vi "FL24 Combi Tool Main.vi"() -> ()   [LabVIEW 2016]
uses:
  Common/LabVIEW GEA2 Toolkit/LabVIEW_GEA2_Toolkit.lvlibp/type defs/Data In.ctl
  Common/LabVIEW GEA2 Toolkit/LabVIEW_GEA2_Toolkit.lvlibp/type defs/Source_Destination.ctl
  Common/LabVIEW GEA2 Toolkit/LabVIEW_GEA2_Toolkit.lvlibp/type defs/Data Type.ctl
  Common/LabVIEW GEA2 Toolkit/LabVIEW_GEA2_Toolkit.lvlibp/type defs/ERD Read Data In.ctl
  Laundry Tool 2.0 Support/type defs2/Select _Graph_Brass.ctl
  Laundry Tool 1.0 Support/type defs/ERD_Graph_All.ctl
  Laundry Tool 1.0 Support/type defs/ERD_Graph.ctl
  Laundry Tool 1.0 Support/type defs/Version.ctl
  Laundry Tool 2.0 Support/type defs2/ERD_Always_Show_Brass.ctl
  Laundry Tool 1.0 Support/type defs/Fault_Buffer_Status.ctl
  Laundry Tool 2.0 Support/type defs2/Diagnostics_Table.ctl
  Laundry Tool 1.0 Support/type defs/Cycle_Diag_Buffer_Status.ctl
  Laundry Tool 1.0 Support/type defs/Motor Control.ctl
  Laundry Tool 1.0 Support/type defs/Valves.ctl
  Laundry Tool 2.0 Support/type defs2/Programming_Brass.ctl
  Laundry Tool 2.0 Support/type defs2/Flash_Results.ctl
  Laundry Tool 2.0 Support/type defs2/ERD_Data_Loop_Control_Brass.ctl
  Laundry Tool 2.0 Support/type defs2/ERD_Loop_States_Brass.ctl
  Laundry Tool 2.0 Support/type defs2/DAQ_States_Brass.ctl
  Laundry Tool 2.0 Support/type defs2/Error_Command_Brass.ctl
  Common/GExplorer Support/typedefs/GExplorer_Data_Cluster.ctl
  Laundry Tool 1.0 Support/type defs/Cont_Send_States.ctl
  Laundry Tool 2.0 Support/type defs2/Cont_Send_States_Brass.ctl
  Common/LabVIEW GEA2 Toolkit/LabVIEW_GEA2_Toolkit.lvlibp/type defs/Data Out.ctl
  Common/LabVIEW GEA2 Toolkit/LabVIEW_GEA2_Toolkit.lvlibp/type defs/ERD Write Data In.ctl
  Laundry Tool 2.0 Support/type defs2/ERD_Loop_Control_Command_Brass.ctl
  Laundry Tool 2.0 Support/type defs2/GEA2_Control_Command_Brass.ctl
  Common/LabVIEW GEA2 Toolkit/LabVIEW_GEA2_Toolkit.lvlibp/advanced/GEA2 Message Received Event Handler.vi
  C:/Automation/DLLs/PC Dot Net/GeaCommunication.dll
  Automation/DLLs/PC Dot Net/GeaCommunication.dll
  Common/LabVIEW GEA2 Toolkit/LabVIEW_GEA2_Toolkit.lvlibp
panel:
  in  "Data ON":bool=TRUE
  out "ERD_Always Show":T1
  in  "Stop":bool
  out "Fault Status":bool
  out "Log Rate (ms)":u32
  in  "Tab Control":T2(tab)
  in  "Programming":T3={"Program"=FALSE, "File Path"=path "", "Program Ind"=FALSE, "Result"=9, "Reset Board"=FALSE, "Enter Bootloader"=FALSE} {"Result" items=["ImageRejected", "BoardNotFound", "UnableToGetGeaConfiguration", "WriteToFlashNotAllowed", "ImageDownloadedSuccessfully", "ImagePresent", "WriteToFlashFailed", "EraseFailed", "CrcFailed", ""]}
  in  "Filter Data":bool=TRUE
  in  "Start Send":bool
  in  "Cmd":string
  in  "Filter Log":bool
  in  "Msg Rate (ms)":u32=1000 min=50 step=50
  out "CSV File Log Path":path=path "C:/Users/502129737/Desktop/1"
  in  "Clear":bool
  out "GEA2 Log":string
  in  "Board Index":u8 max=0 step=1
  out "Board ID":string="0"
  in  "GEA2 Send":T5={"Source"=228, "Destination"=60, "Command"=0, "Message"=""} {"Command" format="%02x"; "Destination" format="%02x"; "Source" format="%02x"}
  in  "Send Button":bool
  in  "GEA2 Log Length":i32=100000
  in  "Save Log":bool
  out "Version":T6
  in  "GEA Inputs":T7={"Source"=228, "Destination"=60} {"Destination" format="%.0x"; "Source" format="%.0x"}
  in  "Read ERD List":T8[](array[typedef])=[{"ERD Number"=0, "Data Type"=enum."string"}] {"ERD Number" format="%.0x"}
  out "Read ERD Data Out":cluster{"ERD Number":u16, "Data":string}[](array[cluster]) {"ERD Number" format="%.0x"}
  in  "Read ERD":bool
  in  "Write ERD":bool
  in  "Write ERD List":T10(array[cluster])=[{"ERD Number"=0, "Data Type"=enum."string", "Data"=""}] {"ERD Number" format="%.0x"}
  out "Washer Loads":u16[][](graph)=[[0, 100, 200, 300, 400]]
  in  "ERD Graphing ON":bool
  out "ERD Graph  Ind":T11
  in  "ERD Graph Cntrl":T12={"ERD 3"={"ERD #"=61458, "Data Type"=enum."uint16_t", "Scaler"=100}, "ERD 2"={"ERD #"=61458, "Data Type"=enum."uint16_t", "Scaler"=100}, "ERD 1"={"ERD #"=61458, "Data Type"=enum."uint16_t", "Scaler"=100}} {"ERD 1"."Scaler" min=1; "ERD 1"."ERD #" format="%.0x"; "ERD 2"."Scaler" min=1; "ERD 2"."ERD #" format="%.0x"; "ERD 3"."Scaler" min=1; "ERD 3"."ERD #" format="%.0x"}
  in  "Graphing ON":bool=TRUE
  in  "Select Graph":T14
  out "ERD 3":dbl(graph)
  out "ERD 2":dbl(graph)
  out "ERD 1":dbl(graph)
  out "Water Temperature":dbl(graph)
  out "Basket Speed":u16(graph)
  out "Pressure 2":dbl(graph)
  out "Dryer Loads":dbl[][](graph)
  in  "Save Fault Log":bool
  in  "Clear Fault Table Buffer":bool
  in  "Clear Fault Seq Buffer":bool
  in  "Fault ON":bool
  out "Fault Table Buffer":string[][](table)
  out "Fault Sequence Buffer":string
  out "Seq Buffer Status":T15
  out "Table Buffer Status":T15
  in  "Save Cycle History Log":bool
  in  "Clear Cycle Buffer":bool
  out "Cycle Buffer Status":T16
  in  "Get Cycle History":bool
  out "Diagnostics Table":T17
  in  "Buzzer":cluster{"Test":bool}
  in  "Drain Pump":cluster{"ON":bool, "OFF":bool}
  in  "Valve Control":T18
  in  "Motor Control":T19={"Speed (RPM)"=50, "Start Motor"=FALSE, "Stop Motor"=FALSE} {"Speed (RPM)" min=-100 max=1400 step=50}
  in  "Test Mode":cluster{"Exit":bool, "Enter":bool}
  in  "Door Lock":cluster{"Lock Door":bool, "Unlock Door":bool}
  in  "LEDs":cluster{"ON":bool, "OFF":bool}
  in  "Drum Light":cluster{"ON":bool, "OFF":bool}
  in  "Water Heater":cluster{"ON":bool, "OFF":bool}
  in  "Dry Heater":cluster{"ON":bool, "OFF":bool}
  in  "ERD Read List":T20(array[cluster])=[{"Boolean"=TRUE, "ERD Number"=1, "ERD Name"="Model Number", "Data Type"=enum."string"}, {"Boolean"=TRUE, "ERD Number"=2, "ERD Name"="Serial Number", "Data Type"=enum."string"}, {"Boolean"=TRUE, "ERD Number"=8192, "ERD Name"="Machine Status", "Data Type"=enum."uint8_t"}, {"Boolean"=TRUE, "ERD Number"=8202, "ERD Name"="Cycle Name", "Data Type"=enum."string"}, {"Boolean"=TRUE, "ERD Number"=8213, "ERD Name"="Soil Level", "Data Type"=enum."string"}, {"Boolean"=TRUE, "ERD Number"=142, "ERD Name"="Cycle Count", "Data Type"=enum."uint32_t"}, {"Boolean"=TRUE, "ERD Number"=8193, "ERD Name"="Sub-Cycle", "Data Type"=enum."string"}, {"Boolean"=TRUE, "ERD Number"=141, "ERD Name"="System Runtime", "Data Type"=enum."uint32_t"}, {"Boolean"=TRUE, "ERD Number"=8208, "ERD Name"="Delay Time", "Data Type"=enum."uint16_t"}, {"Boolean"=TRUE, "ERD Number"=70, "ERD Name"="Cycle Time", "Data Type"=enum."uint16_t"}, {"Boolean"=TRUE, "ERD Number"=8206, "ERD Name"="Operating Mode", "Data Type"=enum."string"}, {"Boolean"=TRUE, "ERD Number"=8214, "ERD Name"="Temp Level", "Data Type"=enum."uint8_t"}, {"Boolean"=TRUE, "ERD Number"=8215, "ERD Name"="Spin Level", "Data Type"=enum."uint8_t"}, {"Boolean"=TRUE, "ERD Number"=61440, "ERD Name"="Water Level", "Data Type"=enum."uint8_t"}, {"Boolean"=TRUE, "ERD Number"=8216, "ERD Name"="Rinse Option", "Data Type"=enum."uint8_t"}, {"Boolean"=TRUE, "ERD Number"=4, "ERD Name"="Control Lock", "Data Type"=enum."string"}, {"Boolean"=TRUE, "ERD Number"=10, "ERD Name"="Signal Volume", "Data Type"=enum."string"}, {"Boolean"=TRUE, "ERD Number"=8236, "ERD Name"="Basket Speed", "Data Type"=enum."uint16_t"}, {"Boolean"=TRUE, "ERD Number"=8210, "ERD Name"="Door Status", "Data Type"=enum."string"}, {"Boolean"=TRUE, "ERD Number"=8211, "ERD Name"="Lock Status", "Data Type"=enum."string"}, {"Boolean"=TRUE, "ERD Number"=8258, "ERD Name"="Pressure (inches)", "Data Type"=enum."uint32_t"}, {"Boolean"=TRUE, "ERD Number"=8259, "ERD Name"="Water Temperature", "Data Type"=enum."uint16_t"}, {"Boolean"=TRUE, "ERD Number"=61458, "ERD Name"="Pressure Hz", "Data Type"=enum."uint16_t"}, {"Boolean"=TRUE, "ERD Number"=61455, "ERD Name"="Load Status 2", "Data Type"=enum."uint8_t"}, {"Boolean"=TRUE, "ERD Number"=61456, "ERD Name"="Load Status 1", "Data Type"=enum."uint8_t"}, {"Boolean"=TRUE, "ERD Number"=61460, "ERD Name"="Firmware Version", "Data Type"=enum."string"}, {"Boolean"=TRUE, "ERD Number"=61452, "ERD Name"="Drum Light", "Data Type"=enum."string"}, {"Boolean"=TRUE, "ERD Number"=14, "ERD Name"="Voltage", "Data Type"=enum."uint16_t"}, {"Boolean"=TRUE, "ERD Number"=61461, "ERD Name"="Inlet Thermistor", "Data Type"=enum."uint16_t"}, {"Boolean"=TRUE, "ERD Number"=61462, "ERD Name"="Outlet Themistor", "Data Type"=enum."uint16_t"}, {"Boolean"=TRUE, "ERD Number"=8275, "ERD Name"="Extended Tumble", "Data Type"=enum."string"}, {"Boolean"=TRUE, "ERD Number"=8277, "ERD Name"="Time Saver", "Data Type"=enum."string"}] {"ERD Number" format="%.0x"}
  out "Error Out":errorcluster
  in  "Error In":errorcluster
  # "UI: 0x3C\nMC: 0x21"
  # "Software Version"
  # "UI - Critical Version"
  # "UI - Non-Critical"
  # "MC -  Version"
  # "Inverter Version"
  # "Model Setting"
  # "Must input a valid ERD# and Data Type\nDO NOT Leave Blank \nIf no scaler use value of 01"
  # "+ CCW   - CW"
  # "Contact:\n\nDerek Hibdon\nderek.hibdon@ge.com"
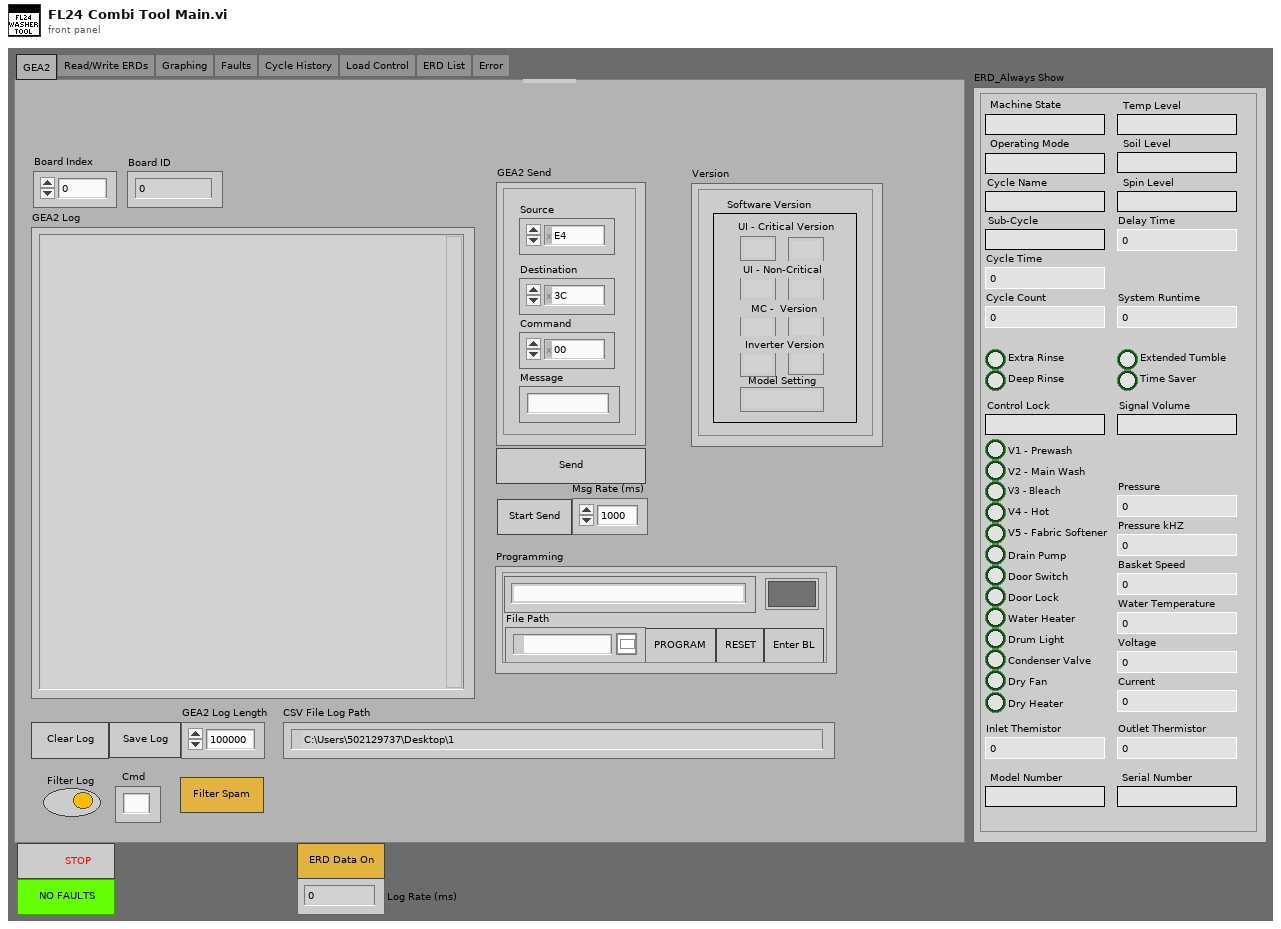
[diagram p1: front panel]
types:
  T1 = typedef "ERD_Always_Show_Brass.ctl" = cluster{"Machine State":string, "Cycle Count":u32, "Soil Level":string, "Spin Level":string, "Temp Level":string, "Delay Time":u16, "Sub-Cycle":string, "Cycle Name":string, "Model Number":string, "Serial Number":string, "System Runtime":u32, "Cycle Time":u16, "Operating Mode":string, "Deep Rinse":bool, "Extra Rinse":bool, "V1 - Prewash":bool, "V2 - Main Wash":bool, "V3 - Bleach":bool, "V4 - Hot":bool, "Drain Pump":bool, "Door Switch":bool, "Door Lock":bool, "Basket Speed":u16, "Water Temperature":dbl, "Voltage":dbl, "Pressure":dbl, "Water Heater":bool, "Control Lock":string, "Signal Volume":string, "Current":u16, "Pressure kHZ":dbl, "Drum Light":bool, "V5 - Fabric Softener":bool, "Inlet Themistor":dbl, "Outlet Thermistor":dbl, "Condenser Valve":bool, "Dry Fan":bool, "Dry Heater":bool, "Extended Tumble":bool, "Time Saver":bool}
  T2 = enum32{"GEA2", "Read/Write ERDs", "Graphing", "Faults", "Cycle History", "Load Control", "ERD List", "Error"}
  T3 = typedef "Programming_Brass.ctl" = cluster{"Program":bool, "File Path":path, "Program Ind":bool, "Result":T4, "Reset Board":bool, "Enter Bootloader":bool}
  T4 = typedef "Flash_Results.ctl" = i32
  T5 = typedef "LabVIEW_GEA2_Toolkit.lvlibp/Data In.ctl" = cluster{"Source":u8, "Destination":u8, "Command":u8, "Message":string}
  T6 = typedef "Version.ctl" = cluster{"UI - Critical Major":string, "UI - Critical Minor":string, "UI - Non-Critical Minor":string, "UI - Non-Critical Major":string, "MC Minor":string, "MC Major":string, "Model Setting":string, "Inverter Version  Minor":string, "Inverter Version Major":string}
  T7 = typedef "LabVIEW_GEA2_Toolkit.lvlibp/Source_Destination.ctl" = cluster{"Source":u8, "Destination":u8}
  T8 = typedef "LabVIEW_GEA2_Toolkit.lvlibp/ERD Read Data In.ctl" = cluster{"ERD Number":u16, "Data Type":T9}
  T9 = typedef "LabVIEW_GEA2_Toolkit.lvlibp/Data Type.ctl" = enum16{"string", "boolean", "uint8_t", "uint16_t", "uint32_t", "uint64_t", "int8_t", "int16_t", "int32_t", "int64_t"}
  T10 = cluster{"ERD Number":u16, "Data Type":T9, "Data":string}[]
  T11 = cluster{"ERD Value 1":dbl, "ERD Value 2":dbl, "ERD Value 3":dbl}
  T12 = typedef "ERD_Graph_All.ctl" = cluster{"ERD 3":T13, "ERD 2":T13, "ERD 1":T13}
  T13 = typedef "ERD_Graph.ctl" = cluster{"ERD #":u16, "Data Type":T9, "Scaler":u32}
  T14 = typedef "Select _Graph_Brass.ctl" = enum16{"Washer Loads", "Dryer Loads", "ERD 1", "ERD 2", "ERD 3", "Water Temperature (F)", "Basket Speed (RPM)", "Pressure (in H2O)"}
  T15 = typedef "Fault_Buffer_Status.ctl" = cluster{"Current Index":u16, "Count":u16, "Overwrite Count":u16}
  T16 = typedef "Cycle_Diag_Buffer_Status.ctl" = cluster{"Current Index":u16, "Count":u16, "Overwrite Count":u16}
  T17 = typedef "Diagnostics_Table.ctl" = string[][]
  T18 = typedef "Valves.ctl" = cluster{"PreWash Valve":bool, "Bleach Valve":bool, "Hot Valve":bool, "Valves ON":bool, "Valves OFF":bool, "MainWash Valve":bool, "Fabric Softener":bool, "Condenser Valve":bool}
  T19 = typedef "Motor Control.ctl" = cluster{"Speed (RPM)":i16, "Start Motor":bool, "Stop Motor":bool}
  T20 = cluster{"Boolean":bool, "ERD Number":u16, "ERD Name":string, "Data Type":enum16{"string", "boolean", "uint8_t", "uint16_t", "uint32_t", "uint64_t"}}[]
  T21 = typedef "Cont_Send_States_Brass.ctl" = enum16{"Run", "Shutdown"}
  T22 = typedef "Cont_Send_States.ctl" = enum16{"Run", "Shutdown"}
  T23 = typedef "GExplorer_Data_Cluster.ctl" = cluster{"Data":variant, "State":enum16{"Add to Log", "Clear", "Shutdown"}}
  T24 = typedef "ERD_Data_Loop_Control_Brass.ctl" = cluster{"Data":variant, "State":T25}
  T25 = typedef "ERD_Loop_States_Brass.ctl" = enum16{"Init", "Build ERD Read List", "Read ERDs", "Update UI", "Update Graphs", "Read Faults", "Log Data", "Pause", "Shutdown"}
  T26 = typedef "Error_Command_Brass.ctl" = enum16{"Initialize", "Handle Errors", "Report Errors"}
  T27 = typedef "DAQ_States_Brass.ctl" = enum16{"Wait for Init", "Rename Devices", "Verify Hardware", "Initialize", "Run", "Shutdown", "Exit"}
  T28 = typedef "LabVIEW_GEA2_Toolkit.lvlibp/ERD Write Data In.ctl" = cluster{"ERD Number":u16, "Data Type":T9, "Data":string}
  T29 = enum8{"Enabled", "Disabled", "Disabled and Grayed Out"}
  T30 = typedef "GEA2_Control_Command_Brass.ctl" = enum16{"Initialize", "Shutdown"}
  T31 = typedef "ERD_Loop_Control_Command_Brass.ctl" = enum16{"Initialize", "Shutdown"}
  T32 = typedef "LabVIEW_GEA2_Toolkit.lvlibp/Data Out.ctl" = cluster{"Source":u8, "Destination":u8, "Command":u8, "Length":u8, "CRC":u16, "Message":string}
  T33 = typedef "LabVIEW_GEA2_Toolkit.lvlibp/ERD Read Data Out.ctl" = cluster{"ERD Number":u16, "Data":string}
  T34 = typedef "All_Bundled_Data_Brass.ctl" = cluster{"Version":T6, "ERD_Always Show":T1, "Personality Set":u8, "CSV File String Arrays":T35, "Fault Table Array ":T36}
  T35 = typedef "CSV_File_String_Arrays.ctl" = cluster{"ERD Number Array":string[], "ERD Name Array":string[], "ERD Converted String Data":string[]}
  T36 = typedef "Fault Table Array.ctl" = T37[]
  T37 = typedef "Fault_Table_Info.ctl" = cluster{"Cycle Count":u32, " Runtime (min) ":u32, "Fault Status":string, "Fault ID":string, "Fault Count":u16}
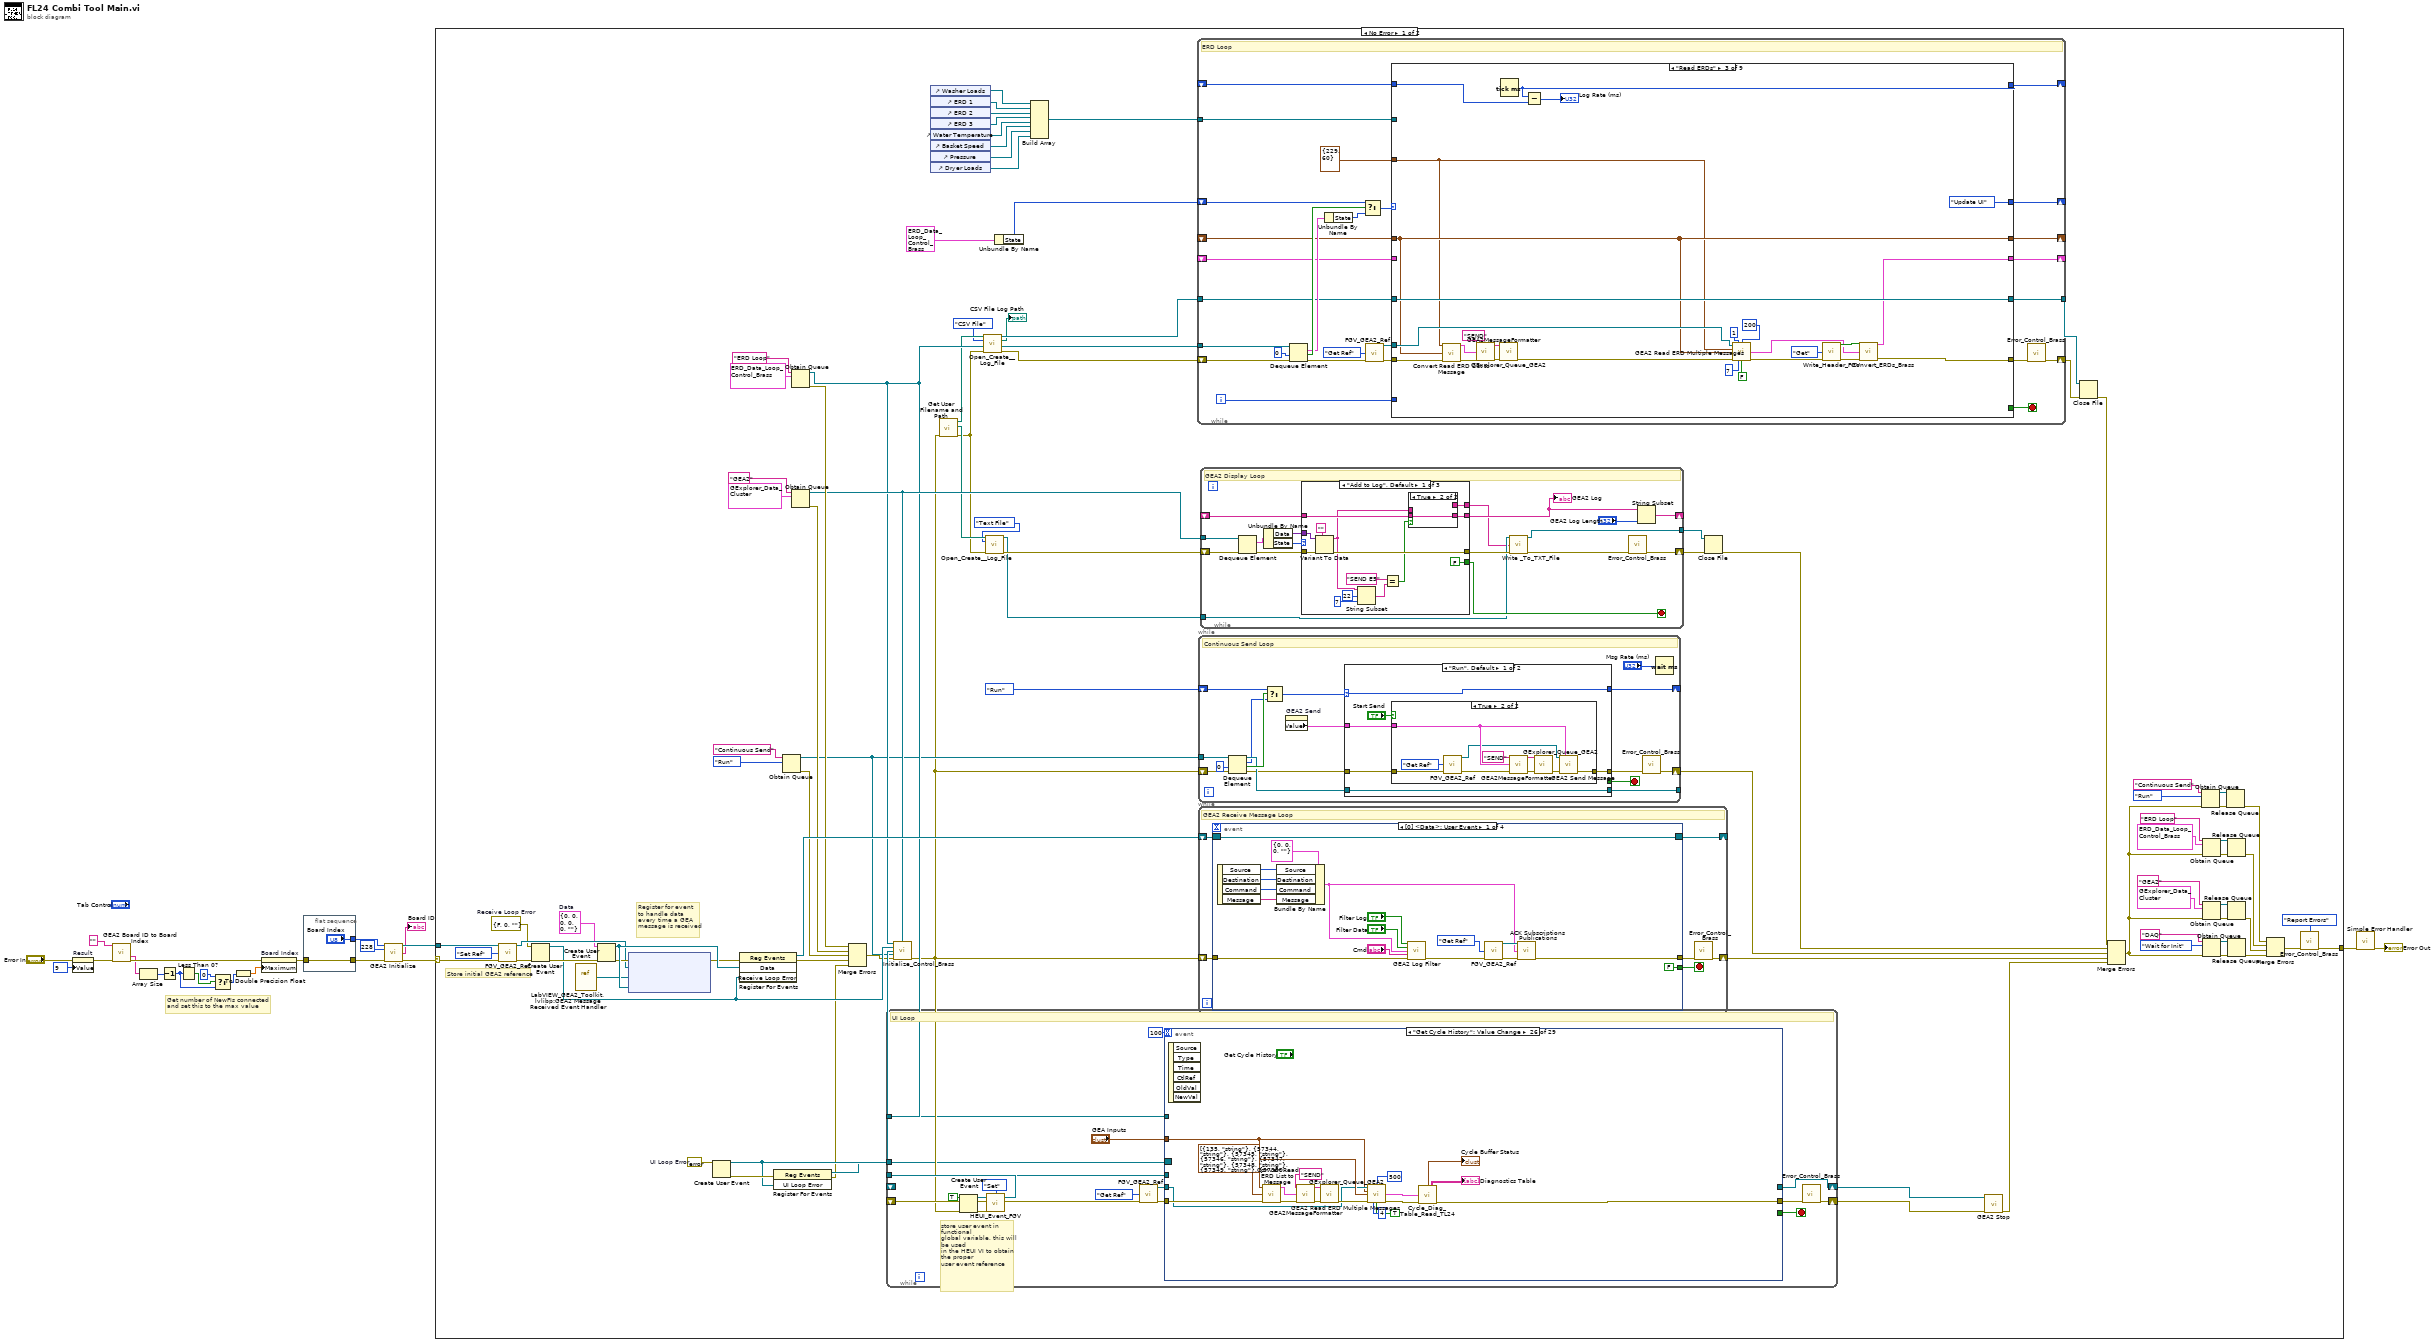
[diagram p0: block diagram]
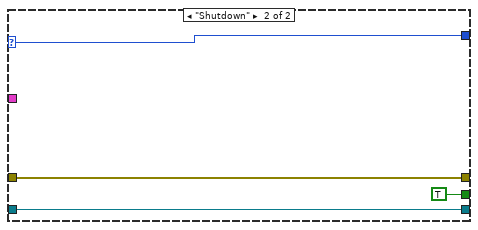
[diagram p3: hidden frame]
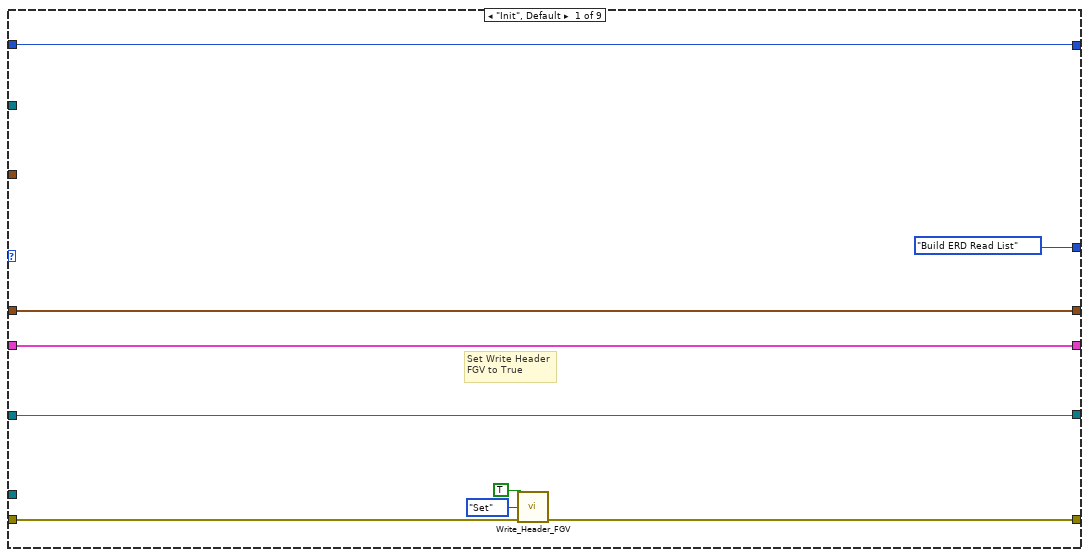
[diagram p4: hidden frame]
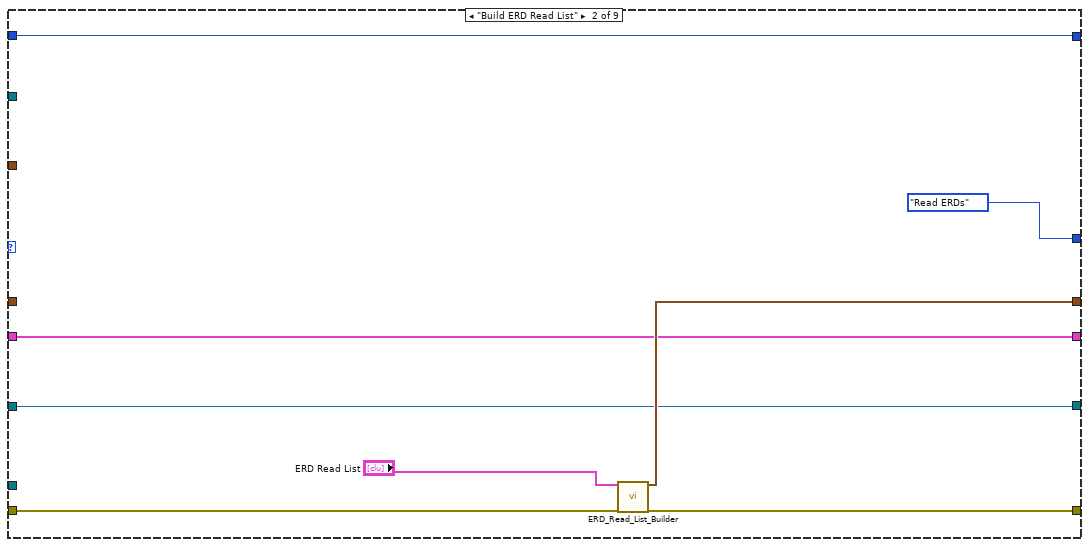
[diagram p5: hidden frame]
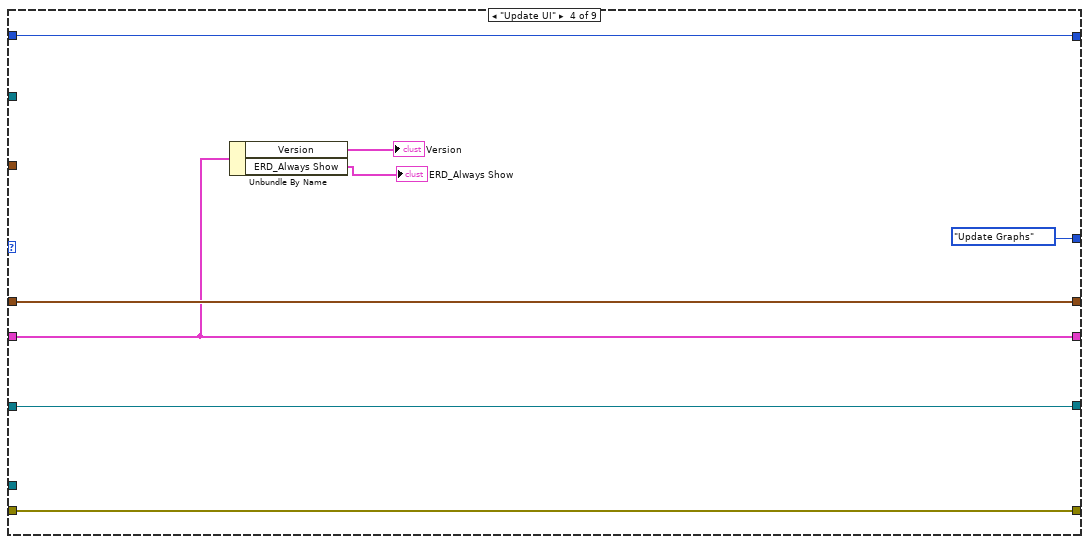
[diagram p6: hidden frame]
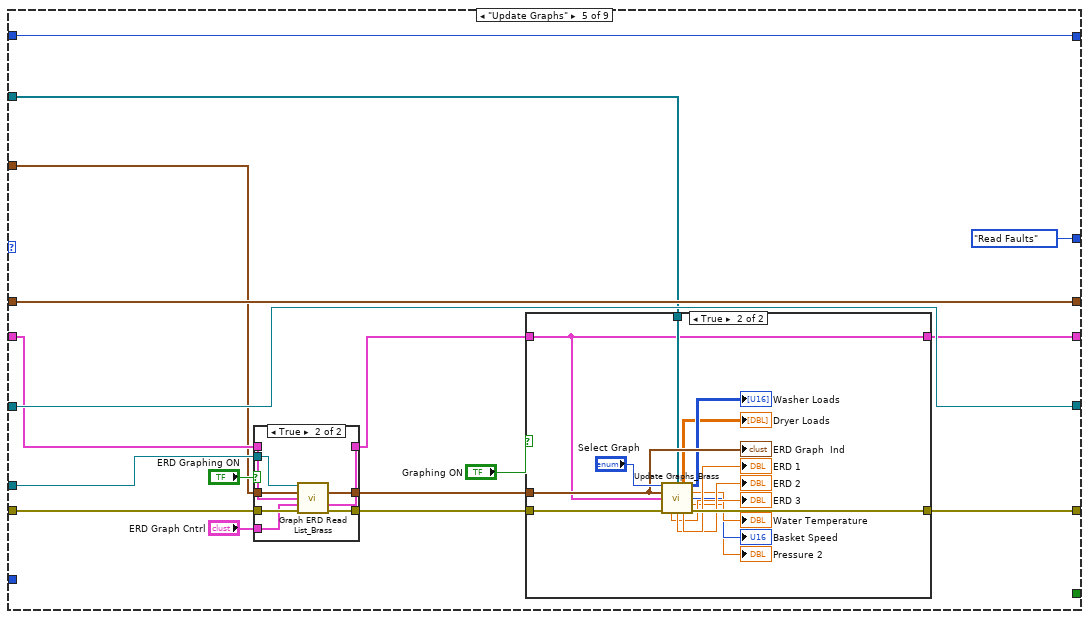
[diagram p7: hidden frame]
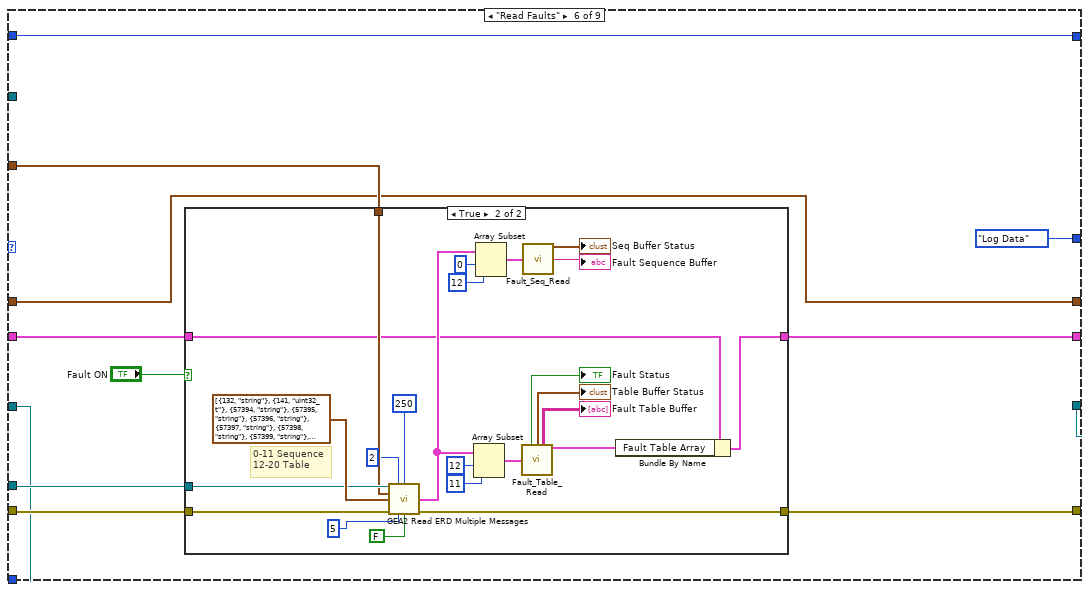
[diagram p10: hidden frame]
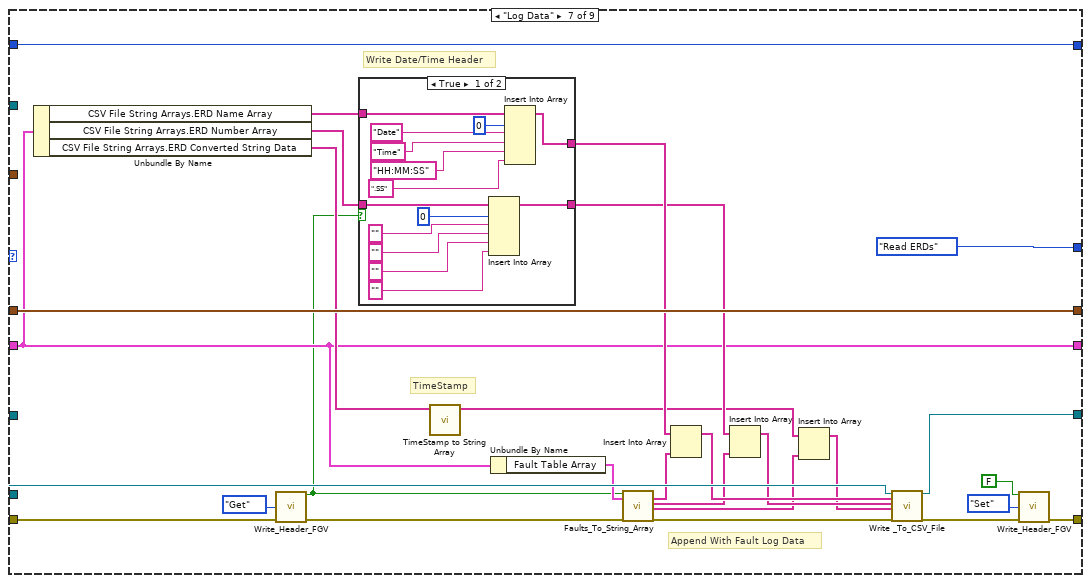
[diagram p12: hidden frame]
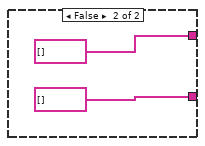
[diagram p13: hidden frame]
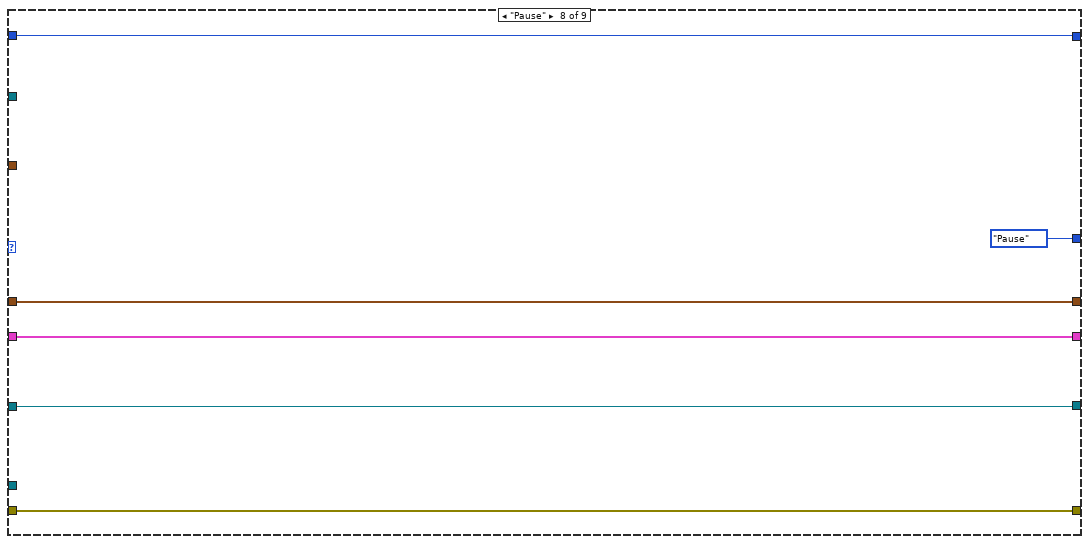
[diagram p14: hidden frame]
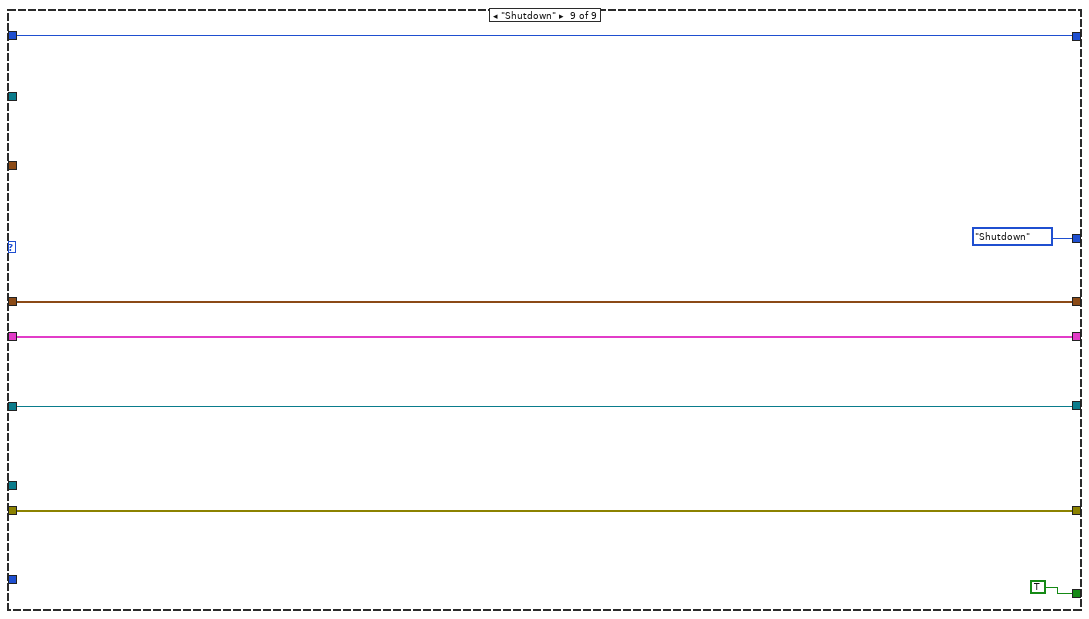
[diagram p15: hidden frame]
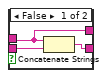
[diagram p16: hidden frame]
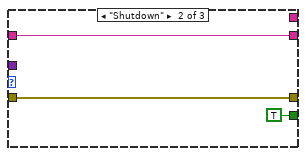
[diagram p17: hidden frame]
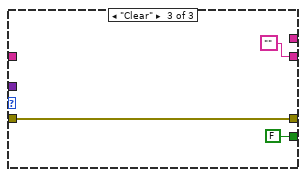
[diagram p18: hidden frame]
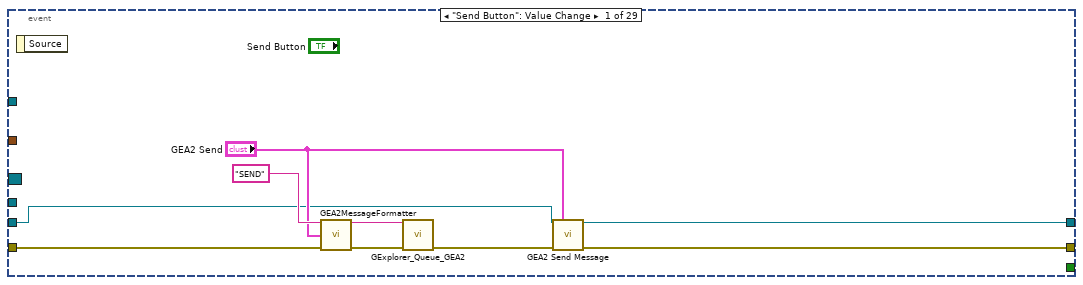
[diagram p19: hidden frame]
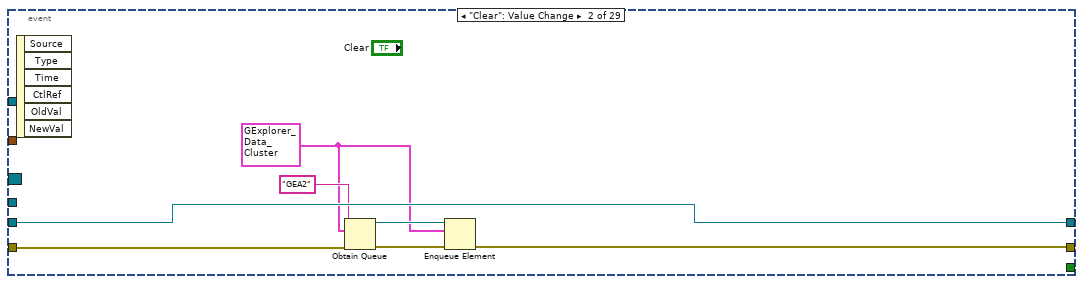
[diagram p20: hidden frame]
diagram:
  w1 = T4 9 items=["ImageRejected", "BoardNotFound", "UnableToGetGeaConfiguration", "WriteToFlashNotAllowed", "ImageDownloadedSuccessfully", "ImagePresent", "WriteToFlashFailed", "EraseFailed", "CrcFailed", ""] ("Value")
  # "Get number of NewFIs connected\nand set this to the max value"
  n1 = property on="Result" class="Ring (strict)"(error in="Error In", "Value"=w1) -> (error out=w2:errorcluster)  [unwired: 1 in, 1 out]
  n2 = call "GEA2 Board ID to Board Index.vi"("Board ID"="", "Error In"=w2) -> ("Boards Found"=w7:string[], "Error Out"=w15:errorcluster)  [unwired: 9 in, 3 out]
  n3 = Array Size(array=w7) -> (size(s)=w12:i32)
  n4 = Decrement(x=w12) -> (x-1=w10:i32)
  n5 = Less Than 0?(x=w10) -> (x < 0?=w11:bool)
  n6 = Select(t=0, s=w11, f=w10) -> (s? t:f=w8:i32)
  n7 = To Double Precision Float(number=w8) -> (double precision float=w6:dbl)
  n8 = property on="Board Index" class="DigNum (strict)"(error in=w15, "Maximum"=w6) -> (error out=w14:errorcluster)  [unwired: 1 in, 1 out]
  n9 = flat-sequence {
    tunnel: ["Board Index"] -> w18
    tunnel: w14 -> [w22]
    tunnel: [w22] -> w13
    frame #0 {
    }
  }
  n10 = call "GEA2 Initialize.vi"("Board Index"=w18, "Source Address"=u8 228, "error in"=w13) -> ("GEA2 Reference Out"=w20:refnum<k24>, "Board ID"=→"Board ID":string, "error out"=w19:errorcluster)  [unwired: 10 in]
  n11 = case shown="No Error" w19 {
    selector: w19 -> [w78 w1223]
    tunnel: w20 -> [w76 _]
    tunnel: [w79 w1223] -> w5
    frame No Error {
      w41 = errorcluster {"status"=FALSE, "code"=0, "source"=""}  # Receive Loop Error
      w42 = T32 {"Source"=0, "Destination"=0, "Command"=0, "Length"=0, "CRC"=0, "Message"=""}  # Data
      w110 = errorcluster {"status"=FALSE, "code"=0, "source"=""}  # UI Loop Error
      # "store user event in functional\nglobal variable, this will be used\nin the HEUI VI to obtain the proper\nuser event reference"
      # "Store initial GEA2 reference"
      # "Register for event\nto handle data\nevery time a GEA\nmessage is received"
      n12 = call "FGV_GEA2_Ref.vi"("GEA2 Reference In"=w76, "Action"=enum16{"Set Ref", "Get Ref"}."Set Ref", "Error In"=w78) -> ("GEA2 Reference Out"=w75:refnum<k24>, "Error Out"=w77:errorcluster)  [unwired: 11 in]
      n13 = Create User Event(user event datatype=w41, error in=w77) -> (user event=w111:refnum<user-event>, error out=w113:errorcluster)
      n14 = vi-ref "LabVIEW_GEA2_Toolkit.lvlibp:GEA2 Message Received Event Handler.vi"() -> (w112:refnum<vi>)
      n15 = Create User Event(user event datatype=w42, error in=w113) -> (user event=w116:refnum<user-event>, error out=w115:errorcluster)
      n16 = node(w115, w75, w112, w116) -> (w114:errorcluster)  [unwired: 1 in, 1 out]
      n17 = Create User Event(user event datatype=w110) -> (user event=w100:refnum<user-event>, error out=w109:errorcluster)  [unwired: 1 in]
      n18 = register-events(error in=w114, w116, w111) -> (reference out=w108:refnum<event-registration>, error out=w83:errorcluster)  [unwired: 1 in]
      n19 = register-events(error in=w109, w100) -> (reference out=w91:refnum<event-registration>, error out=w82:errorcluster)  [unwired: 1 in]
      n20 = Obtain Queue(name (unnamed)="Continuous Send", element data type=Cont_Send_States_Brass."Run" ("State")) -> (queue out=w43:refnum<queue>, error out=w48:errorcluster)  [unwired: 3 in, 1 out]
      n21 = Obtain Queue(name (unnamed)="ERD Loop", element data type=T24 {"Data"=variant, "State"=enum."Read ERDs"} ("Data")) -> (queue out=w63:refnum<queue>, error out=w80:errorcluster)  [unwired: 3 in, 1 out]
      n22 = Obtain Queue(name (unnamed)="GEA2", element data type=T23 {"Data"=variant, "State"=enum."Add to Log"} ("Data")) -> (queue out=w64:refnum<queue>, error out=w84:errorcluster)  [unwired: 3 in, 1 out]
      n23 = Merge Errors(w80, w84, w48, w83, w82) -> (w81:errorcluster)
      n24 = call "Initialize_Control_Brass.vi"("ERD Loop"=w63, "GEA2"=w64, "Receive Loop"=w111, "UI Loop Error"=w100, "Cont Send"=w43, "Error In"=w81) -> ("Error Out"=w38:errorcluster)  [unwired: 9 in]
      n25 = control-ref of="Washer Loads"() -> (w28:refnum<vi>)
      n26 = control-ref of="ERD 1"() -> (w61:refnum<vi>)
      n27 = control-ref of="ERD 2"() -> (w59:refnum<vi>)
      n28 = control-ref of="ERD 3"() -> (w60:refnum<vi>)
      n29 = control-ref of="Water Temperature"() -> (w27:refnum<vi>)
      n30 = control-ref of="Basket Speed"() -> (w26:refnum<vi>)
      n31 = control-ref of="Pressure"() -> (w25:refnum<vi>)
      n32 = control-ref of="Dryer Loads"() -> (w24:refnum<vi>)
      n33 = call "Get User Filename and Path.vi"("error in (no error)"=w38) -> ("error out"=w30:errorcluster, "TXT File Path"=w36:path, "CSV File Path"=w39:path)  [unwired: 8 in]
      n34 = Create User Event(user event datatype=TRUE ("Bool"), error in=w38) -> (user event=w70:refnum<user-event>, error out=w71:errorcluster)
      n35 = call "Open_Create__Log_File.vi"("File Path Control"=w39, "Enum"=enum16{"CSV File", "Text File"}."CSV File", "Error In"=w30) -> ("refnum out"=w62:refnum<file>, "File Path"=→"CSV File Log Path":path, "Error Out"=w73:errorcluster)  [unwired: 10 in]
      n36 = call "Open_Create__Log_File.vi"("File Path Control"=w36, "Enum"=enum16{"CSV File", "Text File"}."Text File", "Error In"=w30) -> ("refnum out"=w35:refnum<file>, "Error Out"=w37:errorcluster)  [unwired: 10 in, 1 out]
      n37 = call "HEUI_Event_FGV.vi"("Event In"=w70, "Action"=enum16{"Get", "Set"}."Set", "Error In"=w71) -> ("Event Out"=w67:refnum<user-event>, "Error Out"=w68:errorcluster)  [unwired: 11 in]
      n38 = while "UI Loop" {
        shift-right: [w424] -> w118
        shift-left: w68 -> [w418]
        shift-right: [w426] -> w117
        shift-left: _ -> [_]
        tunnel: w91 -> [w425]
        tunnel: w67 -> [w415]
        tunnel: w63 -> [w414]
        stop <- w423 stop-if-true
        # "UI Loop"
        n39 = call "FGV_GEA2_Ref.vi"("Action"=enum16{"Set Ref", "Get Ref"}."Get Ref", "Error In"=w418) -> ("GEA2 Reference Out"=w417:refnum<k24>, "Error Out"=w419:errorcluster)  [unwired: 12 in]
        n40 = event shown="[25] \"Get Cycle History\": Value Change" {
          selector: w425 -> [_ _ _ _ _ _ _ _ _ _ _ _ _ _ _ _ _ _ _ _ _ _ _ _ _ _ _ _ _]
          dyn-events: _ -> [_ _ _ _ _ _ _ _ _ _ _ _ _ _ _ _ _ _ _ _ _ _ _ _ _ _ _ _ _]
          timeout: 100 -> [_ _ _ _ _ _ _ _ _ _ _ _ _ _ _ _ _ _ _ _ _ _ _ _ _ _ _ _ _]
          tunnel: [w432 w442 w443 w449 w463 w473 w486 w493 w496 w515 w530 w574 w618 w662 w699 w782 w821 w860 w874 w918 w962 w989 w1033 w1083 w1102 w1116 w1134 w1154 w1165] -> w422
          tunnel: w419 -> [w429 w439 w443 w445 w460 w477 w484 w491 w500 w518 w534 w578 w622 w666 w703 w794 w839 w868 w878 w922 w966 w993 w1038 w1086 w1108 w1124 w1140 w1155 w1171]
          tunnel: [_ _ _ _ _ _ _ _ _ _ _ _ _ _ _ _ _ _ _ _ _ _ _ _ _ _ _ _ TRUE] -> w423
          tunnel: w417 -> [w427 w441 w444 w447 w461 _ _ _ w502 w517 w533 w577 w621 w665 w702 w785 w838 w867 w877 w921 w965 w992 w1037 w1085 w1107 w1118 w1139 _ w1174]
          tunnel: [w434 w441 w444 w450 w462 _ _ _ _ w516 _ _ _ _ _ w784 _ _ _ _ _ _ _ w1084 _ _ _ _ w1174] -> w426
          tunnel: "GEA Inputs" -> [_ _ _ w448 w458 _ _ _ w501 w519 w532 w576 w620 w664 w701 w786 w834 w865 w876 w920 w964 w991 w1036 w1087 w1105 w1117 w1141 _ _]
          tunnel: w415 -> [_ _ _ _ _ _ _ _ _ _ _ _ _ _ _ _ _ _ _ _ _ _ _ _ _ _ _ _ _]
          tunnel: w414 -> [_ _ _ _ _ _ w482 w489 _ _ _ _ _ _ _ w781 _ w858 _ _ _ _ _ _ _ _ _ w1152 _]
          event "Send Button": Value Change {
            n41 = event-data() -> ()  [unwired: 1 in, 1 out]
            n42 = call "GEA2MessageFormatter.vi"("Prefix(Send/Recv)"="SEND", "GEA2 Data In"="GEA2 Send", "Error In"=w429) -> ("Output String"=w431:string, "Error Out"=w430:errorcluster)  [unwired: 11 in]
            n43 = call "GExplorer_Queue_GEA2.vi"("Output String"=w431, "error in (no error)"=w430) -> ("error out"=w433:errorcluster)  [unwired: 13 in]
            n44 = call "GEA2 Send Message.vi"("GEA2 Reference In"=w427, "Input Data"="GEA2 Send", "Error In"=w433) -> ("GEA2 Reference Out"=w434:refnum<k24>, "Error Out"=w432:errorcluster)  [unwired: 11 in]
          }
          event "Clear": Value Change {
            w436 = T23 {"Data"=variant, "State"=enum."Clear"} ("element")
            n45 = event-data() -> ()  [unwired: 1 in, 6 out]
            n46 = Obtain Queue(name (unnamed)="GEA2", element data type=w436, error in (no error)=w439) -> (queue out=w437:refnum<queue>, error out=w440:errorcluster)  [unwired: 2 in, 1 out]
            n47 = Enqueue Element(queue=w437, element=w436, error in (no error)=w440) -> (error out=w442:errorcluster)  [unwired: 1 in, 2 out]
          }
          event Timeout {
            # "Must have timeout case to give GEA2 FGV a chance to update\nthe GEA2 reference. Otherwise, when we receive an event it may\nbe using a reference that is no longer valid."
            n48 = event-data() -> ()  [unwired: 1 in, 3 out]
          }
          event "Write ERD": Value Change {
            n49 = event-data() -> ()  [unwired: 1 in, 1 out]
            n50 = call "Convert Write ERD List to Message.vi"("GEA Inputs"=w448, "Write ERD List"="Write ERD List", "Error In"=w445) -> ("GEA Message"=w454:T5, "Error Out"=w455:errorcluster)  [unwired: 11 in]
            n51 = call "GEA2MessageFormatter.vi"("Prefix(Send/Recv)"="SEND", "GEA2 Data In"=w454, "Error In"=w455) -> ("Output String"=w456:string, "Error Out"=w457:errorcluster)  [unwired: 11 in]
            n52 = call "GExplorer_Queue_GEA2.vi"("Output String"=w456, "error in (no error)"=w457) -> ("error out"=w452:errorcluster)  [unwired: 13 in]
            n53 = call "GEA2 Write ERD.vi"("GEA2 Reference In"=w447, "GEA Inputs"=w448, "Write ERD List"="Write ERD List", "Error In"=w452, "Verify ERD Response?"=FALSE) -> ("GEA2 Reference Out"=w450:refnum<k24>, "Error Out"=w449:errorcluster)  [unwired: 8 in, 1 out]
          }
          event "Read ERD": Value Change {
            n54 = event-data() -> ()  [unwired: 1 in, 6 out]
            n55 = call "Convert Read ERD List to Message.vi"("GEA Inputs"=w458, "Read ERD List"="Read ERD List", "Error In"=w460) -> ("GEA Message"=w468:T5, "Error Out"=w459:errorcluster)  [unwired: 11 in]
            n56 = call "GEA2MessageFormatter.vi"("Prefix(Send/Recv)"="SEND", "GEA2 Data In"=w468, "Error In"=w459) -> ("Output String"=w466:string, "Error Out"=w465:errorcluster)  [unwired: 11 in]
            n57 = call "GExplorer_Queue_GEA2.vi"("Output String"=w466, "error in (no error)"=w465) -> ("error out"=w469:errorcluster)  [unwired: 13 in]
            n58 = call "GEA2 Read ERD.vi"("GEA2 Reference In"=w461, "GEA Inputs"=w458, "Read ERD List"="Read ERD List", "Error In"=w469, "Verify ERD Response?"=FALSE) -> ("GEA2 Reference Out"=w462:refnum<k24>, "ERD Data Out"=→"Read ERD Data Out":T33[], "Error Out"=w463:errorcluster)  [unwired: 7 in, 1 out]
          }
          event "Save Log": Value Change {
            n59 = event-data() -> ()  [unwired: 1 in, 6 out]
            n60 = property on="GEA2 Log" class="Str"(error in=w477) -> (error out=w479:errorcluster, "Value"=w478:string)  [unwired: 1 in, 1 out]
            n61 = Write to Text File(prompt (Choose or enter file path)="Choose filename and path to save txt file to ", text=w478, error in=w479) -> (refnum out=w476:refnum<file>, error out=w475:errorcluster)  [unwired: 1 in, 1 out]
            n62 = Close File(refnum=w476, error in=w475) -> (error out=w474:errorcluster)  [unwired: 1 out]
            n63 = call <vilib>:"Clear Errors.vi"("error in (no error)"=w474, "specific error code to clear (0: all)"=43) -> ("error out"=w473:errorcluster)  [unwired: 4 in, 1 out]
          }
          event "ERD Read List": Value Change {
            n64 = event-data() -> ()  [unwired: 1 in, 6 out]
            n65 = Enqueue Element(queue=w482, element=T24 {"Data"=variant, "State"=enum."Build ERD Read List"}, error in (no error)=w484) -> (error out=w483:errorcluster)  [unwired: 1 in, 2 out]
            n66 = call "Write_Header_FGV.vi"("Write Header ? In"=TRUE, "Action"=enum16{"Get", "Set"}."Set", "Error In"=w483) -> ("Error Out"=w486:errorcluster)  [unwired: 11 in, 1 out]
          }
          event "Fault ON", "ERD Graphing ON": Value Change {
            n67 = event-data() -> ()  [unwired: 1 in, 6 out]
            n68 = Enqueue Element(queue=w489, element=T24 {"Data"=variant, "State"=enum."Build ERD Read List"}, error in (no error)=w491) -> (error out=w490:errorcluster)  [unwired: 1 in, 2 out]
            n69 = call "Write_Header_FGV.vi"("Write Header ? In"=TRUE, "Action"=enum16{"Get", "Set"}."Set", "Error In"=w490) -> ("Error Out"=w493:errorcluster)  [unwired: 11 in, 1 out]
          }
          event "Save Fault Log": Value Change {
            # "0-16 Sequence\n17-27 Table"
            n70 = event-data() -> ()  [unwired: 1 in, 6 out]
            n71 = call "GEA2 Read ERD Multiple Messages.vi"("GEA2 Reference In"=w502, "Read Timeout (ms)"=u32 250, "GEA Inputs"=w501, "Read ERD List"=T8[] [{"ERD Number"=132, "Data Type"=enum."string"}, {"ERD Number"=141, "Data Type"=enum."uint32_t"}, {"ERD Number"=57394, "Data Type"=enum."string"}, {"ERD Number"=57395, "Data Type"=enum."string"}, {"ERD Number"=57396, "Data Type"=enum."string"}, {"ERD Number"=57397, "Data Type"=enum."string"}, {"ERD Number"=57398, "Data Type"=enum."string"}, {"ERD Number"=57399, "Data Type"=enum."string"}, {"ERD Number"=57400, "Data Type"=enum."string"}, {"ERD Number"=57401, "Data Type"=enum."string"}, {"ERD Number"=57402, "Data Type"=enum."string"}, {"ERD Number"=57403, "Data Type"=enum."string"}, {"ERD Number"=57404, "Data Type"=enum."string"}, {"ERD Number"=57405, "Data Type"=enum."string"}, {"ERD Number"=57406, "Data Type"=enum."string"}, {"ERD Number"=57407, "Data Type"=enum."string"}, {"ERD Number"=57408, "Data Type"=enum."string"}, {"ERD Number"=129, "Data Type"=enum."string"}, {"ERD Number"=57444, "Data Type"=enum."string"}, {"ERD Number"=57445, "Data Type"=enum."string"}, {"ERD Number"=57446, "Data Type"=enum."string"}, {"ERD Number"=57447, "Data Type"=enum."string"}, {"ERD Number"=57448, "Data Type"=enum."string"}, {"ERD Number"=57449, "Data Type"=enum."string"}, {"ERD Number"=57450, "Data Type"=enum."string"}, {"ERD Number"=57451, "Data Type"=enum."string"}, {"ERD Number"=57452, "Data Type"=enum."string"}, {"ERD Number"=57453, "Data Type"=enum."string"}], "Error In"=w500, "#ERDs per message"=14 ("#ERDs per message 2"), "Verify ERD Response?"=FALSE) -> ("ERD Data Out"=w505:T33[], "Error Out"=w497:errorcluster)  [unwired: 5 in, 2 out]
            n72 = Array Subset(array=w505, index=17, length=10) -> (w506:T33[])
            n73 = Array Subset(array=w505, index=0, length=17) -> (w504:T33[])
            n74 = call "Fault_Seq_Read.vi"("Seq ERD In"=w504) -> ("String"=w499:string)  [unwired: 13 in, 1 out]
            n75 = call "Fault_Table_Read.vi"("ERD Data Out"=w506) -> ("Fault Table String Out"=w498:string[][])  [unwired: 11 in, 3 out]
            n76 = call "Fault_Logging.vi"("String"=w499, "Fault Table String Out"=w498, "error in (no error)"=w497) -> ("error out"=w496:errorcluster)  [unwired: 12 in]
          }
          event "Clear Fault Seq Buffer": Value Change {
            n77 = event-data() -> ()  [unwired: 1 in, 6 out]
            n78 = Bundle By Name(cluster=T28 {"ERD Number"=133, "Data Type"=enum."string", "Data"=""} ("ERD Read Data In"), "Data"="FF") -> (w528:T28)
            n79 = Build Array(w528) -> (w522:T28[])
            n80 = call "Convert Write ERD List to Message.vi"("GEA Inputs"=w519, "Write ERD List"=w522, "Error In"=w518) -> ("GEA Message"=w524:T5, "Error Out"=w525:errorcluster)  [unwired: 11 in]
            n81 = call "GEA2MessageFormatter.vi"("Prefix(Send/Recv)"="SEND", "GEA2 Data In"=w524, "Error In"=w525) -> ("Output String"=w526:string, "Error Out"=w527:errorcluster)  [unwired: 11 in]
            n82 = call "GExplorer_Queue_GEA2.vi"("Output String"=w526, "error in (no error)"=w527) -> ("error out"=w523:errorcluster)  [unwired: 13 in]
            n83 = call "GEA2 Write ERD.vi"("GEA2 Reference In"=w517, "Read Timeout (ms)"=u32 2000, "GEA Inputs"=w519, "Write ERD List"=w522, "Error In"=w523, "Verify ERD Response?"=FALSE) -> ("GEA2 Reference Out"=w516:refnum<k24>, "Error Out"=w515:errorcluster)  [unwired: 7 in, 1 out]
          }
          event "Door Lock.Lock Door", "Door Lock.Unlock Door": Value Change {
            n84 = event-data() -> ("CtlRef"=w531:refnum<vi>)  [unwired: 1 in, 5 out]
            n85 = property class="Bool"(reference=w531, error in=w534) -> (reference out=w537:refnum<vi>, error out=w538:errorcluster, "Label.Text"=w539:string)
            n86 = Close Reference(reference=w537, error in (no error)=w538) -> (error out=w536:errorcluster)
            n87 = case shown="\"Lock Door\"" w539 {
              tunnel: [w544 w570] -> w530
              tunnel: w533 -> [w545 w569]
              tunnel: w536 -> [w546 w561]
              tunnel: w532 -> [w543 w560]
              tunnel: [w542 w559] -> _
              tunnel: T28 {"ERD Number"=61441, "Data Type"=enum."string", "Data"=""} ("ERD Read Data In") -> [w540 w557]
              frame "Unlock Door", Default {
                n88 = Concatenate Strings("00" ("string")) -> (w556:string)
                n89 = Bundle By Name(cluster=w540, "Data"=w556) -> (w555:T28)
                n90 = Build Array(w555) -> (w548:T28[])
                n91 = call "Convert Write ERD List to Message.vi"("GEA Inputs"=w543, "Write ERD List"=w548, "Error In"=w546) -> ("GEA Message"=w550:T5, "Error Out"=w551:errorcluster)  [unwired: 11 in]
                n92 = call "GEA2MessageFormatter.vi"("Prefix(Send/Recv)"="SEND", "GEA2 Data In"=w550, "Error In"=w551) -> ("Output String"=w552:string, "Error Out"=w553:errorcluster)  [unwired: 11 in]
                n93 = call "GExplorer_Queue_GEA2.vi"("Output String"=w552, "error in (no error)"=w553) -> ("error out"=w549:errorcluster)  [unwired: 13 in]
                n94 = call "GEA2 Write ERD.vi"("GEA2 Reference In"=w545, "GEA Inputs"=w543, "Write ERD List"=w548, "Error In"=w549, "Verify ERD Response?"=TRUE) -> ("GEA2 Reference Out"=w542:refnum<k24>, "Error Out"=w544:errorcluster)  [unwired: 8 in, 1 out]
              }
              frame "Lock Door" {
                n95 = Concatenate Strings("01" ("string")) -> (w573:string)
                n96 = Bundle By Name(cluster=w557, "Data"=w573) -> (w572:T28)
                n97 = Build Array(w572) -> (w563:T28[])
                n98 = call "Convert Write ERD List to Message.vi"("GEA Inputs"=w560, "Write ERD List"=w563, "Error In"=w561) -> ("GEA Message"=w565:T5, "Error Out"=w566:errorcluster)  [unwired: 11 in]
                n99 = call "GEA2MessageFormatter.vi"("Prefix(Send/Recv)"="SEND", "GEA2 Data In"=w565, "Error In"=w566) -> ("Output String"=w567:string, "Error Out"=w568:errorcluster)  [unwired: 11 in]
                n100 = call "GExplorer_Queue_GEA2.vi"("Output String"=w567, "error in (no error)"=w568) -> ("error out"=w564:errorcluster)  [unwired: 13 in]
                n101 = call "GEA2 Write ERD.vi"("GEA2 Reference In"=w569, "GEA Inputs"=w560, "Write ERD List"=w563, "Error In"=w564, "Verify ERD Response?"=TRUE) -> ("GEA2 Reference Out"=w559:refnum<k24>, "Error Out"=w570:errorcluster)  [unwired: 8 in, 1 out]
              }
            }
          }
          event "Drain Pump.ON", "Drain Pump.OFF": Value Change {
            n102 = event-data() -> ("CtlRef"=w575:refnum<vi>)  [unwired: 1 in, 5 out]
            n103 = property class="Bool"(reference=w575, error in=w578) -> (reference out=w581:refnum<vi>, error out=w582:errorcluster, "Label.Text"=w583:string)
            n104 = Close Reference(reference=w581, error in (no error)=w582) -> (error out=w580:errorcluster)
            n105 = case shown="\"ON\"" w583 {
              tunnel: [w588 w614] -> w574
              tunnel: w577 -> [w589 w613]
              tunnel: w580 -> [w590 w605]
              tunnel: w576 -> [w587 w604]
              tunnel: [w586 w603] -> _
              tunnel: T28 {"ERD Number"=61451, "Data Type"=enum."string", "Data"=""} ("ERD Read Data In") -> [w584 w601]
              frame "OFF", Default {
                n106 = Concatenate Strings("00" ("string")) -> (w600:string)
                n107 = Bundle By Name(cluster=w584, "Data"=w600) -> (w599:T28)
                n108 = Build Array(w599) -> (w592:T28[])
                n109 = call "Convert Write ERD List to Message.vi"("GEA Inputs"=w587, "Write ERD List"=w592, "Error In"=w590) -> ("GEA Message"=w594:T5, "Error Out"=w595:errorcluster)  [unwired: 11 in]
                n110 = call "GEA2MessageFormatter.vi"("Prefix(Send/Recv)"="SEND", "GEA2 Data In"=w594, "Error In"=w595) -> ("Output String"=w596:string, "Error Out"=w597:errorcluster)  [unwired: 11 in]
                n111 = call "GExplorer_Queue_GEA2.vi"("Output String"=w596, "error in (no error)"=w597) -> ("error out"=w593:errorcluster)  [unwired: 13 in]
                n112 = call "GEA2 Write ERD.vi"("GEA2 Reference In"=w589, "GEA Inputs"=w587, "Write ERD List"=w592, "Error In"=w593, "Verify ERD Response?"=TRUE) -> ("GEA2 Reference Out"=w586:refnum<k24>, "Error Out"=w588:errorcluster)  [unwired: 8 in, 1 out]
              }
              frame "ON" {
                n113 = Concatenate Strings("08" ("string")) -> (w617:string)
                n114 = Bundle By Name(cluster=w601, "Data"=w617) -> (w616:T28)
                n115 = Build Array(w616) -> (w607:T28[])
                n116 = call "Convert Write ERD List to Message.vi"("GEA Inputs"=w604, "Write ERD List"=w607, "Error In"=w605) -> ("GEA Message"=w609:T5, "Error Out"=w610:errorcluster)  [unwired: 11 in]
                n117 = call "GEA2MessageFormatter.vi"("Prefix(Send/Recv)"="SEND", "GEA2 Data In"=w609, "Error In"=w610) -> ("Output String"=w611:string, "Error Out"=w612:errorcluster)  [unwired: 11 in]
                n118 = call "GExplorer_Queue_GEA2.vi"("Output String"=w611, "error in (no error)"=w612) -> ("error out"=w608:errorcluster)  [unwired: 13 in]
                n119 = call "GEA2 Write ERD.vi"("GEA2 Reference In"=w613, "GEA Inputs"=w604, "Write ERD List"=w607, "Error In"=w608, "Verify ERD Response?"=TRUE) -> ("GEA2 Reference Out"=w603:refnum<k24>, "Error Out"=w614:errorcluster)  [unwired: 8 in, 1 out]
              }
            }
          }
          event "Water Heater.ON", "Water Heater.OFF": Value Change {
            n120 = event-data() -> ("CtlRef"=w619:refnum<vi>)  [unwired: 1 in, 5 out]
            n121 = property class="Bool"(reference=w619, error in=w622) -> (reference out=w625:refnum<vi>, error out=w626:errorcluster, "Label.Text"=w627:string)
            n122 = Close Reference(reference=w625, error in (no error)=w626) -> (error out=w624:errorcluster)
            n123 = case shown="\"ON\"" w627 {
              tunnel: [w632 w658] -> w618
              tunnel: w621 -> [w633 w657]
              tunnel: w624 -> [w634 w649]
              tunnel: w620 -> [w631 w648]
              tunnel: [w630 w647] -> _
              tunnel: T28 {"ERD Number"=61450, "Data Type"=enum."string", "Data"=""} ("ERD Read Data In") -> [w628 w645]
              frame "OFF", Default {
                n124 = Concatenate Strings("00" ("string")) -> (w644:string)
                n125 = Bundle By Name(cluster=w628, "Data"=w644) -> (w643:T28)
                n126 = Build Array(w643) -> (w636:T28[])
                n127 = call "Convert Write ERD List to Message.vi"("GEA Inputs"=w631, "Write ERD List"=w636, "Error In"=w634) -> ("GEA Message"=w638:T5, "Error Out"=w639:errorcluster)  [unwired: 11 in]
                n128 = call "GEA2MessageFormatter.vi"("Prefix(Send/Recv)"="SEND", "GEA2 Data In"=w638, "Error In"=w639) -> ("Output String"=w640:string, "Error Out"=w641:errorcluster)  [unwired: 11 in]
                n129 = call "GExplorer_Queue_GEA2.vi"("Output String"=w640, "error in (no error)"=w641) -> ("error out"=w637:errorcluster)  [unwired: 13 in]
                n130 = call "GEA2 Write ERD.vi"("GEA2 Reference In"=w633, "GEA Inputs"=w631, "Write ERD List"=w636, "Error In"=w637, "Verify ERD Response?"=TRUE) -> ("GEA2 Reference Out"=w630:refnum<k24>, "Error Out"=w632:errorcluster)  [unwired: 8 in, 1 out]
              }
              frame "ON" {
                n131 = Concatenate Strings("02" ("string")) -> (w661:string)
                n132 = Bundle By Name(cluster=w645, "Data"=w661) -> (w660:T28)
                n133 = Build Array(w660) -> (w651:T28[])
                n134 = call "Convert Write ERD List to Message.vi"("GEA Inputs"=w648, "Write ERD List"=w651, "Error In"=w649) -> ("GEA Message"=w653:T5, "Error Out"=w654:errorcluster)  [unwired: 11 in]
                n135 = call "GEA2MessageFormatter.vi"("Prefix(Send/Recv)"="SEND", "GEA2 Data In"=w653, "Error In"=w654) -> ("Output String"=w655:string, "Error Out"=w656:errorcluster)  [unwired: 11 in]
                n136 = call "GExplorer_Queue_GEA2.vi"("Output String"=w655, "error in (no error)"=w656) -> ("error out"=w652:errorcluster)  [unwired: 13 in]
                n137 = call "GEA2 Write ERD.vi"("GEA2 Reference In"=w657, "GEA Inputs"=w648, "Write ERD List"=w651, "Error In"=w652, "Verify ERD Response?"=TRUE) -> ("GEA2 Reference Out"=w647:refnum<k24>, "Error Out"=w658:errorcluster)  [unwired: 8 in, 1 out]
              }
            }
          }
          event "Dry Heater.ON", "Dry Heater.OFF": Value Change {
            n138 = event-data() -> ("CtlRef"=w663:refnum<vi>)  [unwired: 1 in, 5 out]
            n139 = property class="Bool"(reference=w663, error in=w666) -> (reference out=w668:refnum<vi>, error out=w669:errorcluster, "Label.Text"=w670:string)
            n140 = Close Reference(reference=w668, error in (no error)=w669) -> (error out=w667:errorcluster)
            n141 = case shown="\"ON\"" w670 {
              tunnel: [w675 w696] -> w662
              tunnel: w665 -> [w676 w695]
              tunnel: w667 -> [w677 w688]
              tunnel: w664 -> [w674 w687]
              tunnel: [w673 w686] -> _
              frame "OFF", Default {
                w671 = T28[] [{"ERD Number"=61450, "Data Type"=enum."string", "Data"="00"}, {"ERD Number"=61444, "Data Type"=enum."string", "Data"=" 0000"}, {"ERD Number"=61451, "Data Type"=enum."string", "Data"="00"}] ("appended array")
                n142 = call "Convert Write ERD List to Message.vi"("GEA Inputs"=w674, "Write ERD List"=w671, "Error In"=w677) -> ("GEA Message"=w680:T5, "Error Out"=w681:errorcluster)  [unwired: 11 in]
                n143 = call "GEA2MessageFormatter.vi"("Prefix(Send/Recv)"="SEND", "GEA2 Data In"=w680, "Error In"=w681) -> ("Output String"=w682:string, "Error Out"=w683:errorcluster)  [unwired: 11 in]
                n144 = call "GExplorer_Queue_GEA2.vi"("Output String"=w682, "error in (no error)"=w683) -> ("error out"=w679:errorcluster)  [unwired: 13 in]
                n145 = call "GEA2 Write ERD.vi"("GEA2 Reference In"=w676, "GEA Inputs"=w674, "Write ERD List"=w671, "Error In"=w679, "Verify ERD Response?"=TRUE) -> ("GEA2 Reference Out"=w673:refnum<k24>, "Error Out"=w675:errorcluster)  [unwired: 8 in, 1 out]
              }
              frame "ON" {
                w684 = T28[] [{"ERD Number"=61450, "Data Type"=enum."string", "Data"="80"}, {"ERD Number"=61444, "Data Type"=enum."string", "Data"="0032"}, {"ERD Number"=61451, "Data Type"=enum."string", "Data"="10"}] ("appended array")
                n146 = call "Convert Write ERD List to Message.vi"("GEA Inputs"=w687, "Write ERD List"=w684, "Error In"=w688) -> ("GEA Message"=w691:T5, "Error Out"=w692:errorcluster)  [unwired: 11 in]
                n147 = call "GEA2MessageFormatter.vi"("Prefix(Send/Recv)"="SEND", "GEA2 Data In"=w691, "Error In"=w692) -> ("Output String"=w693:string, "Error Out"=w694:errorcluster)  [unwired: 11 in]
                n148 = call "GExplorer_Queue_GEA2.vi"("Output String"=w693, "error in (no error)"=w694) -> ("error out"=w690:errorcluster)  [unwired: 13 in]
                n149 = call "GEA2 Write ERD.vi"("GEA2 Reference In"=w695, "GEA Inputs"=w687, "Write ERD List"=w684, "Error In"=w690, "Verify ERD Response?"=TRUE) -> ("GEA2 Reference Out"=w686:refnum<k24>, "Error Out"=w696:errorcluster)  [unwired: 8 in, 1 out]
              }
            }
          }
          event Value Change {
            n150 = event-data() -> ("CtlRef"=w700:refnum<vi>)  [unwired: 1 in, 5 out]
            n151 = property class="Bool"(reference=w700, error in=w703) -> (reference out=w706:refnum<vi>, error out=w707:errorcluster, "Label.Text"=w708:string)
            n152 = Close Reference(reference=w706, error in (no error)=w707) -> (error out=w705:errorcluster)
            n153 = case shown="\"Valves OFF\", Default" w708 {
              tunnel: [w723 w766] -> w699
              tunnel: w702 -> [w724 w765]
              tunnel: w705 -> [w725 w757]
              tunnel: w701 -> [w722 w756]
              tunnel: [w721 w755] -> _
              tunnel: T28 {"ERD Number"=61451, "Data Type"=enum."string", "Data"=""} ("ERD Read Data In") -> [w719 w753]
              tunnel: T28 {"ERD Number"=61450, "Data Type"=enum."string", "Data"=""} ("ERD Read Data In") -> [w716 w739]
              tunnel: "Valve Control" -> [_ w752]
              frame "Valves OFF", Default {
                n154 = Concatenate Strings("00" ("string")) -> (w717:string)
                n155 = Concatenate Strings("00" ("string")) -> (w735:string)
                n156 = Bundle By Name(cluster=w716, "Data"=w717) -> (w715:T28)
                n157 = Bundle By Name(cluster=w719, "Data"=w735) -> (w734:T28)
                n158 = Build Array(w734, w715) -> (w727:T28[])
                n159 = call "Convert Write ERD List to Message.vi"("GEA Inputs"=w722, "Write ERD List"=w727, "Error In"=w725) -> ("GEA Message"=w729:T5, "Error Out"=w730:errorcluster)  [unwired: 11 in]
                n160 = property on="Bleach Valve" class="Bool (strict)"("Value"=FALSE) -> ()  [unwired: 2 in, 2 out]
                n161 = property on="PreWash Valve" class="Bool (strict)"("Value"=FALSE) -> ()  [unwired: 2 in, 2 out]
                n162 = call "GEA2MessageFormatter.vi"("Prefix(Send/Recv)"="SEND", "GEA2 Data In"=w729, "Error In"=w730) -> ("Output String"=w731:string, "Error Out"=w732:errorcluster)  [unwired: 11 in]
                n163 = property on="Hot Valve" class="Bool (strict)"("Value"=FALSE) -> ()  [unwired: 2 in, 2 out]
                n164 = property on="MainWash Valve" class="Bool (strict)"("Value"=FALSE) -> ()  [unwired: 2 in, 2 out]
                n165 = call "GExplorer_Queue_GEA2.vi"("Output String"=w731, "error in (no error)"=w732) -> ("error out"=w728:errorcluster)  [unwired: 13 in]
                n166 = call "GEA2 Write ERD.vi"("GEA2 Reference In"=w724, "GEA Inputs"=w722, "Write ERD List"=w727, "Error In"=w728, "Verify ERD Response?"=TRUE) -> ("GEA2 Reference Out"=w721:refnum<k24>, "Error Out"=w723:errorcluster)  [unwired: 8 in, 1 out]
                n167 = property on="Condenser Valve" class="Bool (strict)"("Value"=FALSE) -> ()  [unwired: 2 in, 2 out]
                n168 = property on="Fabric Softener" class="Bool (strict)"("Value"=FALSE) -> ()  [unwired: 2 in, 2 out]
              }
              frame "Valves ON" {
                n169 = Unbundle By Name(w752) -> ("Fabric Softener"=w737:bool, "PreWash Valve"=w738:bool, "MainWash Valve"=w751:bool, "Bleach Valve"=w750:bool, "Hot Valve"=w744:bool, "Condenser Valve"=w736:bool)
                n170 = case shown="False" w737 {
                  tunnel: w751 -> [w774 w779]
                  tunnel: w750 -> [w773 _]
                  tunnel: [w772 w780] -> w749
                  tunnel: w738 -> [w771 _]
                  tunnel: w736 -> [w770 w776]
                  frame False {
                    w769 = FALSE
                    n171 = Build Array(w771, w774, w773, w769, w769, w769, w769, w770) -> (w772:bool[])
                  }
                  frame True {
                    w775 = FALSE
                    n172 = Build Array(TRUE ("element"), w779, TRUE ("element"), w775, w775, w775, w775, w776) -> (w780:bool[])
                  }
                }
                n173 = Select(t="20", s=w744, f="00") -> (s? t:f=w741:string)
                n174 = Boolean Array To Number(Boolean array=w749) -> (number=w748:u32)
                n175 = Number To Hexadecimal String(1:i16 2 ("width (-)"), 2:w748) -> (0:w746:string)
                n176 = Concatenate Strings(w746) -> (w768:string)
                n177 = Concatenate Strings(w741) -> (w745:string)
                n178 = Bundle By Name(cluster=w753, "Data"=w768) -> (w767:T28)
                n179 = Bundle By Name(cluster=w739, "Data"=w745) -> (w740:T28)
                n180 = Build Array(w767, w740) -> (w759:T28[])
                n181 = call "Convert Write ERD List to Message.vi"("GEA Inputs"=w756, "Write ERD List"=w759, "Error In"=w757) -> ("GEA Message"=w761:T5, "Error Out"=w762:errorcluster)  [unwired: 11 in]
                n182 = call "GEA2MessageFormatter.vi"("Prefix(Send/Recv)"="SEND", "GEA2 Data In"=w761, "Error In"=w762) -> ("Output String"=w763:string, "Error Out"=w764:errorcluster)  [unwired: 11 in]
                n183 = call "GExplorer_Queue_GEA2.vi"("Output String"=w763, "error in (no error)"=w764) -> ("error out"=w760:errorcluster)  [unwired: 13 in]
                n184 = call "GEA2 Write ERD.vi"("GEA2 Reference In"=w765, "GEA Inputs"=w756, "Write ERD List"=w759, "Error In"=w760, "Verify ERD Response?"=TRUE) -> ("GEA2 Reference Out"=w755:refnum<k24>, "Error Out"=w766:errorcluster)  [unwired: 8 in, 1 out]
              }
            }
          }
          event Value Change {
            w793 = TRUE ("Value")
            n185 = event-data() -> ()  [unwired: 1 in, 6 out]
            n186 = property on="Program Ind" class="Bool (strict)"(error in=w794, "Value"=w793, "Blinking"=w793) -> (error out=w792:errorcluster)  [unwired: 1 in, 1 out]
            n187 = Enqueue Element(queue=w781, element=T24 {"Data"=variant, "State"=enum."Pause"}, error in (no error)=w792) -> (error out=w788:errorcluster)  [unwired: 1 in, 2 out]
            n188 = Unbundle By Name("Programming") -> ("File Path"=w783:path)
            n189 = Not Equal?(x=w783, y=path "") -> (x != y?=w787:bool)
            n190 = case shown="True" w787 {
              tunnel: w788 -> [w796 w806]
              tunnel: w786 -> [_ w815]
              tunnel: w785 -> [w795 w812]
              tunnel: [w795 w811] -> w784
              tunnel: w783 -> [_ w810]
              tunnel: [w796 w799] -> w782
              tunnel: w781 -> [_ w798]
              frame False {
              }
              frame True {
                w804 = FALSE ("Value")
                w808 = T4 9 items=["ImageRejected", "BoardNotFound", "UnableToGetGeaConfiguration", "WriteToFlashNotAllowed", "ImageDownloadedSuccessfully", "ImagePresent", "WriteToFlashFailed", "EraseFailed", "CrcFailed", ""] ("Value")
                n191 = Unbundle By Name(w815) -> ("Source"=w814:u8, "Destination"=w813:u8)
                n192 = property on="Result" class="Ring (strict)"(error in=w806, "Value"=w808) -> (error out=w809:errorcluster)  [unwired: 1 in, 1 out]
                n193 = call "GEA2 Flash APL.vi"("GEA2 Reference In"=w812, "Force Update?"=TRUE, "Source Address"=w814, "Destination Address"=w813, "File Path"=w810, "Error In"=w809, "Broadcast"=TRUE, "Reset?"=FALSE ("Reset Board?")) -> ("GEA2 Reference Out"=w811:refnum<k24>, "Result"=w803:i32, "Error Out"=w802:errorcluster)  [unwired: 3 in, 2 out]
                n194 = property on="Board Index" class="DigNum (strict)"(error in=w806, "DisabledEnum"=T29."Disabled and Grayed Out" ("Disabled")) -> ()  [unwired: 1 in, 2 out]
                n195 = property on="Result" class="Ring (strict)"(error in=w802, "Value"=w803) -> (error out=w801:errorcluster)  [unwired: 1 in, 1 out]
                n196 = property on="Program Ind" class="Bool (strict)"(error in=w801, "Value"=w804, "Blinking"=w804) -> (error out=w800:errorcluster)  [unwired: 1 in, 1 out]
                n197 = property on="Board Index" class="DigNum (strict)"(error in=w801, "DisabledEnum"=T29."Enabled" ("Disabled")) -> ()  [unwired: 1 in, 2 out]
                n198 = Enqueue Element(queue=w798, element=T24 {"Data"=variant, "State"=enum."Init"}, error in (no error)=w800) -> (error out=w799:errorcluster)  [unwired: 1 in, 2 out]
              }
            }
          }
          event Value Change {
            n199 = event-data() -> ()  [unwired: 1 in, 6 out]
            n200 = Unbundle By Name(w834) -> ("Source"=w820:u8, "Destination"=w832:u8)
            n201 = Bundle By Name(cluster=T5 {"Source"=228, "Destination"=52, "Command"=221, "Message"="F401"} ("Input Data"), "Source"=w820, "Destination"=w832, "Command"=u8 221, "Message"="07") -> (w833:T5)
            n202 = call "GEA2 Send Message.vi"("GEA2 Reference In"=w838, "Input Data"=w833, "Error In"=w839) -> ("GEA2 Reference Out"=w822:refnum<k24>, "Error Out"=w843:errorcluster)  [unwired: 11 in]
            n203 = call "GEA2MessageFormatter.vi"("Prefix(Send/Recv)"="SEND", "GEA2 Data In"=w833, "Error In"=w843) -> ("Output String"=w841:string, "Error Out"=w840:errorcluster)  [unwired: 11 in]
            n204 = call "GExplorer_Queue_GEA2.vi"("Output String"=w841, "error in (no error)"=w840) -> ("error out"=w823:errorcluster)  [unwired: 13 in]
            n205 = Bundle By Name(cluster=T5 {"Source"=228, "Destination"=60, "Command"=221, "Message"="F401"} ("Input Data"), "Source"=w820, "Destination"=u8 255, "Command"=u8 221, "Message"="07") -> (w824:T5)
            n206 = call "GEA2 Send Message.vi"("GEA2 Reference In"=w822, "Input Data"=w824, "Error In"=w823) -> ("Error Out"=w831:errorcluster)  [unwired: 11 in, 1 out]
            n207 = call "GEA2MessageFormatter.vi"("Prefix(Send/Recv)"="SEND", "GEA2 Data In"=w824, "Error In"=w831) -> ("Output String"=w829:string, "Error Out"=w828:errorcluster)  [unwired: 11 in]
            n208 = call "GExplorer_Queue_GEA2.vi"("Output String"=w829, "error in (no error)"=w828) -> ("error out"=w821:errorcluster)  [unwired: 13 in]
          }
          event Value Change {
            n209 = event-data() -> ()  [unwired: 1 in, 6 out]
            n210 = Unbundle By Name(w865) -> ("Source"=w846:u8, "Destination"=w857:u8)
            n211 = Bundle By Name(cluster=T5 {"Source"=228, "Destination"=52, "Command"=221, "Message"="F401"} ("Input Data"), "Source"=w846, "Destination"=w857, "Command"=u8 221, "Message"="F4 01") -> (w863:T5)
            n212 = call "GEA2 Send Message.vi"("GEA2 Reference In"=w867, "Input Data"=w863, "Error In"=w868) -> ("GEA2 Reference Out"=w844:refnum<k24>, "Error Out"=w873:errorcluster)  [unwired: 11 in]
            n213 = call "GEA2MessageFormatter.vi"("Prefix(Send/Recv)"="SEND", "GEA2 Data In"=w863, "Error In"=w873) -> ("Output String"=w871:string, "Error Out"=w870:errorcluster)  [unwired: 11 in]
            n214 = call "GExplorer_Queue_GEA2.vi"("Output String"=w871, "error in (no error)"=w870) -> ("error out"=w848:errorcluster)  [unwired: 13 in]
            n215 = Bundle By Name(cluster=T5 {"Source"=228, "Destination"=52, "Command"=221, "Message"="F401"} ("Input Data"), "Source"=w846, "Destination"=u8 255, "Command"=u8 221, "Message"="F4 01") -> (w855:T5)
            n216 = call "GEA2 Send Message.vi"("GEA2 Reference In"=w844, "Input Data"=w855, "Error In"=w848) -> ("Error Out"=w849:errorcluster)  [unwired: 11 in, 1 out]
            n217 = call "GEA2MessageFormatter.vi"("Prefix(Send/Recv)"="SEND", "GEA2 Data In"=w855, "Error In"=w849) -> ("Output String"=w851:string, "Error Out"=w852:errorcluster)  [unwired: 11 in]
            n218 = call "GExplorer_Queue_GEA2.vi"("Output String"=w851, "error in (no error)"=w852) -> ("error out"=w847:errorcluster)  [unwired: 13 in]
            n219 = call "Time Delay2"("error in (no error)"=w847, "Delay Time (s)"=2.0) -> ("error out"=w861:errorcluster)  [unwired: 9 in]
            n220 = Enqueue Element(queue=w858, element=T24 {"Data"=variant, "State"=enum."Init"} ("Data"), error in (no error)=w861) -> (error out=w860:errorcluster)  [unwired: 1 in, 2 out]
          }
          event "Drum Light.ON", "Drum Light.OFF": Value Change {
            n221 = event-data() -> ("CtlRef"=w875:refnum<vi>)  [unwired: 1 in, 5 out]
            n222 = property class="Bool"(reference=w875, error in=w878) -> (reference out=w881:refnum<vi>, error out=w882:errorcluster, "Label.Text"=w883:string)
            n223 = Close Reference(reference=w881, error in (no error)=w882) -> (error out=w880:errorcluster)
            n224 = case shown="\"OFF\", Default" w883 {
              tunnel: [w888 w914] -> w874
              tunnel: w877 -> [w889 w913]
              tunnel: w880 -> [w890 w905]
              tunnel: w876 -> [w887 w904]
              tunnel: [w886 w903] -> _
              tunnel: T28 {"ERD Number"=61448, "Data Type"=enum."string", "Data"=""} ("ERD Read Data In") -> [w884 w901]
              frame "OFF", Default {
                n225 = Concatenate Strings("00" ("string")) -> (w900:string)
                n226 = Bundle By Name(cluster=w884, "Data"=w900) -> (w899:T28)
                n227 = Build Array(w899) -> (w892:T28[])
                n228 = call "Convert Write ERD List to Message.vi"("GEA Inputs"=w887, "Write ERD List"=w892, "Error In"=w890) -> ("GEA Message"=w894:T5, "Error Out"=w895:errorcluster)  [unwired: 11 in]
                n229 = call "GEA2MessageFormatter.vi"("Prefix(Send/Recv)"="SEND", "GEA2 Data In"=w894, "Error In"=w895) -> ("Output String"=w896:string, "Error Out"=w897:errorcluster)  [unwired: 11 in]
                n230 = call "GExplorer_Queue_GEA2.vi"("Output String"=w896, "error in (no error)"=w897) -> ("error out"=w893:errorcluster)  [unwired: 13 in]
                n231 = call "GEA2 Write ERD.vi"("GEA2 Reference In"=w889, "GEA Inputs"=w887, "Write ERD List"=w892, "Error In"=w893, "Verify ERD Response?"=TRUE) -> ("GEA2 Reference Out"=w886:refnum<k24>, "Error Out"=w888:errorcluster)  [unwired: 8 in, 1 out]
              }
              frame "ON" {
                n232 = Concatenate Strings("01" ("string")) -> (w917:string)
                n233 = Bundle By Name(cluster=w901, "Data"=w917) -> (w916:T28)
                n234 = Build Array(w916) -> (w907:T28[])
                n235 = call "Convert Write ERD List to Message.vi"("GEA Inputs"=w904, "Write ERD List"=w907, "Error In"=w905) -> ("GEA Message"=w909:T5, "Error Out"=w910:errorcluster)  [unwired: 11 in]
                n236 = call "GEA2MessageFormatter.vi"("Prefix(Send/Recv)"="SEND", "GEA2 Data In"=w909, "Error In"=w910) -> ("Output String"=w911:string, "Error Out"=w912:errorcluster)  [unwired: 11 in]
                n237 = call "GExplorer_Queue_GEA2.vi"("Output String"=w911, "error in (no error)"=w912) -> ("error out"=w908:errorcluster)  [unwired: 13 in]
                n238 = call "GEA2 Write ERD.vi"("GEA2 Reference In"=w913, "GEA Inputs"=w904, "Write ERD List"=w907, "Error In"=w908, "Verify ERD Response?"=TRUE) -> ("GEA2 Reference Out"=w903:refnum<k24>, "Error Out"=w914:errorcluster)  [unwired: 8 in, 1 out]
              }
            }
          }
          event "LEDs.ON", "LEDs.OFF": Value Change {
            n239 = event-data() -> ("CtlRef"=w919:refnum<vi>)  [unwired: 1 in, 5 out]
            n240 = property class="Bool"(reference=w919, error in=w922) -> (reference out=w925:refnum<vi>, error out=w926:errorcluster, "Label.Text"=w927:string)
            n241 = Close Reference(reference=w925, error in (no error)=w926) -> (error out=w924:errorcluster)
            n242 = case shown="\"ON\"" w927 {
              tunnel: [w932 w958] -> w918
              tunnel: w921 -> [w933 w957]
              tunnel: w924 -> [w934 w949]
              tunnel: w920 -> [w931 w948]
              tunnel: [w930 w947] -> _
              tunnel: T28 {"ERD Number"=61447, "Data Type"=enum."string", "Data"=""} ("ERD Read Data In") -> [w928 w945]
              frame "OFF", Default {
                n243 = Concatenate Strings("00 00 00 00 00 00 00 00 00 00 00" ("string")) -> (w944:string)
                n244 = Bundle By Name(cluster=w928, "Data"=w944) -> (w943:T28)
                n245 = Build Array(w943) -> (w936:T28[])
                n246 = call "Convert Write ERD List to Message.vi"("GEA Inputs"=w931, "Write ERD List"=w936, "Error In"=w934) -> ("GEA Message"=w938:T5, "Error Out"=w939:errorcluster)  [unwired: 11 in]
                n247 = call "GEA2MessageFormatter.vi"("Prefix(Send/Recv)"="SEND", "GEA2 Data In"=w938, "Error In"=w939) -> ("Output String"=w940:string, "Error Out"=w941:errorcluster)  [unwired: 11 in]
                n248 = call "GExplorer_Queue_GEA2.vi"("Output String"=w940, "error in (no error)"=w941) -> ("error out"=w937:errorcluster)  [unwired: 13 in]
                n249 = call "GEA2 Write ERD.vi"("GEA2 Reference In"=w933, "GEA Inputs"=w931, "Write ERD List"=w936, "Error In"=w937, "Verify ERD Response?"=TRUE) -> ("GEA2 Reference Out"=w930:refnum<k24>, "Error Out"=w932:errorcluster)  [unwired: 8 in, 1 out]
              }
              frame "ON" {
                n250 = Concatenate Strings("FF FF FF FF FF FF FF FF FF FF FF" ("string")) -> (w961:string)
                n251 = Bundle By Name(cluster=w945, "Data"=w961) -> (w960:T28)
                n252 = Build Array(w960) -> (w951:T28[])
                n253 = call "Convert Write ERD List to Message.vi"("GEA Inputs"=w948, "Write ERD List"=w951, "Error In"=w949) -> ("GEA Message"=w953:T5, "Error Out"=w954:errorcluster)  [unwired: 11 in]
                n254 = call "GEA2MessageFormatter.vi"("Prefix(Send/Recv)"="SEND", "GEA2 Data In"=w953, "Error In"=w954) -> ("Output String"=w955:string, "Error Out"=w956:errorcluster)  [unwired: 11 in]
                n255 = call "GExplorer_Queue_GEA2.vi"("Output String"=w955, "error in (no error)"=w956) -> ("error out"=w952:errorcluster)  [unwired: 13 in]
                n256 = call "GEA2 Write ERD.vi"("GEA2 Reference In"=w957, "GEA Inputs"=w948, "Write ERD List"=w951, "Error In"=w952, "Verify ERD Response?"=TRUE) -> ("GEA2 Reference Out"=w947:refnum<k24>, "Error Out"=w958:errorcluster)  [unwired: 8 in, 1 out]
              }
            }
          }
          event "Buzzer.Test": Value Change {
            n257 = event-data() -> ("CtlRef"=w963:refnum<vi>)  [unwired: 1 in, 5 out]
            n258 = property class="Bool"(reference=w963, error in=w966) -> (reference out=w969:refnum<vi>, error out=w970:errorcluster, "Label.Text"=w971:string)
            n259 = Close Reference(reference=w969, error in (no error)=w970) -> (error out=w968:errorcluster)
            n260 = case shown="\"Test\", Default" w971 {
              tunnel: [w976] -> w962
              tunnel: w965 -> [w977]
              tunnel: w968 -> [w978]
              tunnel: w964 -> [w975]
              tunnel: [w974] -> _
              tunnel: T28 {"ERD Number"=61449, "Data Type"=enum."string", "Data"=""} ("ERD Read Data In") -> [w972]
              frame "Test", Default {
                n261 = Concatenate Strings("FF" ("string")) -> (w988:string)
                n262 = Bundle By Name(cluster=w972, "Data"=w988) -> (w987:T28)
                n263 = Build Array(w987) -> (w980:T28[])
                n264 = call "Convert Write ERD List to Message.vi"("GEA Inputs"=w975, "Write ERD List"=w980, "Error In"=w978) -> ("GEA Message"=w982:T5, "Error Out"=w983:errorcluster)  [unwired: 11 in]
                n265 = call "GEA2MessageFormatter.vi"("Prefix(Send/Recv)"="SEND", "GEA2 Data In"=w982, "Error In"=w983) -> ("Output String"=w984:string, "Error Out"=w985:errorcluster)  [unwired: 11 in]
                n266 = call "GExplorer_Queue_GEA2.vi"("Output String"=w984, "error in (no error)"=w985) -> ("error out"=w981:errorcluster)  [unwired: 13 in]
                n267 = call "GEA2 Write ERD.vi"("GEA2 Reference In"=w977, "GEA Inputs"=w975, "Write ERD List"=w980, "Error In"=w981, "Verify ERD Response?"=TRUE) -> ("GEA2 Reference Out"=w974:refnum<k24>, "Error Out"=w976:errorcluster)  [unwired: 8 in, 1 out]
              }
            }
          }
          event "Test Mode.Exit", "Test Mode.Enter": Value Change {
            n268 = event-data() -> ("CtlRef"=w990:refnum<vi>)  [unwired: 1 in, 5 out]
            n269 = property class="Bool"(reference=w990, error in=w993) -> (reference out=w996:refnum<vi>, error out=w997:errorcluster, "Label.Text"=w998:string)
            n270 = Close Reference(reference=w996, error in (no error)=w997) -> (error out=w995:errorcluster)
            n271 = case shown="\"Exit\"" w998 {
              tunnel: [w1003 w1029] -> w989
              tunnel: w992 -> [w1004 w1028]
              tunnel: w995 -> [w1005 w1020]
              tunnel: w991 -> [w1002 w1019]
              tunnel: [w1001 w1018] -> _
              tunnel: T28 {"ERD Number"=61440, "Data Type"=enum."string", "Data"=""} ("ERD Read Data In") -> [w999 w1016]
              frame "Enter", Default {
                n272 = Concatenate Strings("01" ("string")) -> (w1015:string)
                n273 = Bundle By Name(cluster=w999, "Data"=w1015) -> (w1014:T28)
                n274 = Build Array(w1014) -> (w1007:T28[])
                n275 = call "Convert Write ERD List to Message.vi"("GEA Inputs"=w1002, "Write ERD List"=w1007, "Error In"=w1005) -> ("GEA Message"=w1009:T5, "Error Out"=w1010:errorcluster)  [unwired: 11 in]
                n276 = call "GEA2MessageFormatter.vi"("Prefix(Send/Recv)"="SEND", "GEA2 Data In"=w1009, "Error In"=w1010) -> ("Output String"=w1011:string, "Error Out"=w1012:errorcluster)  [unwired: 11 in]
                n277 = call "GExplorer_Queue_GEA2.vi"("Output String"=w1011, "error in (no error)"=w1012) -> ("error out"=w1008:errorcluster)  [unwired: 13 in]
                n278 = call "GEA2 Write ERD.vi"("GEA2 Reference In"=w1004, "GEA Inputs"=w1002, "Write ERD List"=w1007, "Error In"=w1008, "Verify ERD Response?"=TRUE) -> ("GEA2 Reference Out"=w1001:refnum<k24>, "Error Out"=w1003:errorcluster)  [unwired: 8 in, 1 out]
              }
              frame "Exit" {
                n279 = Concatenate Strings("00" ("string")) -> (w1032:string)
                n280 = Bundle By Name(cluster=w1016, "Data"=w1032) -> (w1031:T28)
                n281 = Build Array(w1031) -> (w1022:T28[])
                n282 = call "Convert Write ERD List to Message.vi"("GEA Inputs"=w1019, "Write ERD List"=w1022, "Error In"=w1020) -> ("GEA Message"=w1024:T5, "Error Out"=w1025:errorcluster)  [unwired: 11 in]
                n283 = call "GEA2MessageFormatter.vi"("Prefix(Send/Recv)"="SEND", "GEA2 Data In"=w1024, "Error In"=w1025) -> ("Output String"=w1026:string, "Error Out"=w1027:errorcluster)  [unwired: 11 in]
                n284 = call "GExplorer_Queue_GEA2.vi"("Output String"=w1026, "error in (no error)"=w1027) -> ("error out"=w1023:errorcluster)  [unwired: 13 in]
                n285 = call "GEA2 Write ERD.vi"("GEA2 Reference In"=w1028, "GEA Inputs"=w1019, "Write ERD List"=w1022, "Error In"=w1023, "Verify ERD Response?"=TRUE) -> ("GEA2 Reference Out"=w1018:refnum<k24>, "Error Out"=w1029:errorcluster)  [unwired: 8 in, 1 out]
              }
            }
          }
          event Value Change {
            n286 = event-data() -> ("CtlRef"=w1035:refnum<vi>)  [unwired: 1 in, 5 out]
            n287 = property class="Bool"(reference=w1035, error in=w1038) -> (reference out=w1041:refnum<vi>, error out=w1042:errorcluster, "Label.Text"=w1043:string)
            n288 = Close Reference(reference=w1041, error in (no error)=w1042) -> (error out=w1040:errorcluster)
            n289 = case shown="\"Start Motor\", Default" w1043 {
              tunnel: [w1052 w1077] -> w1033
              tunnel: w1037 -> [w1053 w1076]
              tunnel: w1040 -> [w1054 w1068]
              tunnel: w1036 -> [w1051 w1067]
              tunnel: [w1050 w1066] -> _
              tunnel: T28 {"ERD Number"=61444, "Data Type"=enum."string", "Data"=""} ("ERD Read Data In") -> [w1048 w1064]
              tunnel: "Motor Control" -> [w1047 _]
              frame "Start Motor", Default {
                n290 = Unbundle By Name(w1047) -> ("Speed (RPM)"=w1045:i16)
                n291 = Number To Hexadecimal String(1:i16 4 ("width (-)"), 2:w1045) -> (0:w1046:string)
                n292 = Concatenate Strings(w1046) -> (w1063:string)
                n293 = Bundle By Name(cluster=w1048, "Data"=w1063) -> (w1062:T28)
                n294 = Build Array(w1062) -> (w1056:T28[])
                n295 = call "Convert Write ERD List to Message.vi"("GEA Inputs"=w1051, "Write ERD List"=w1056, "Error In"=w1054) -> ("GEA Message"=w1058:T5, "Error Out"=w1059:errorcluster)  [unwired: 11 in]
                n296 = call "GEA2MessageFormatter.vi"("Prefix(Send/Recv)"="SEND", "GEA2 Data In"=w1058, "Error In"=w1059) -> ("Output String"=w1060:string, "Error Out"=w1061:errorcluster)  [unwired: 11 in]
                n297 = call "GExplorer_Queue_GEA2.vi"("Output String"=w1060, "error in (no error)"=w1061) -> ("error out"=w1057:errorcluster)  [unwired: 13 in]
                n298 = call "GEA2 Write ERD.vi"("GEA2 Reference In"=w1053, "GEA Inputs"=w1051, "Write ERD List"=w1056, "Error In"=w1057, "Verify ERD Response?"=TRUE) -> ("GEA2 Reference Out"=w1050:refnum<k24>, "Error Out"=w1052:errorcluster)  [unwired: 8 in, 1 out]
              }
              frame "Stop Motor" {
                n299 = Concatenate Strings("00 00" ("string")) -> (w1080:string)
                n300 = Bundle By Name(cluster=w1064, "Data"=w1080) -> (w1079:T28)
                n301 = Build Array(w1079) -> (w1070:T28[])
                n302 = call "Convert Write ERD List to Message.vi"("GEA Inputs"=w1067, "Write ERD List"=w1070, "Error In"=w1068) -> ("GEA Message"=w1072:T5, "Error Out"=w1073:errorcluster)  [unwired: 11 in]
                n303 = call "GEA2MessageFormatter.vi"("Prefix(Send/Recv)"="SEND", "GEA2 Data In"=w1072, "Error In"=w1073) -> ("Output String"=w1074:string, "Error Out"=w1075:errorcluster)  [unwired: 11 in]
                n304 = call "GExplorer_Queue_GEA2.vi"("Output String"=w1074, "error in (no error)"=w1075) -> ("error out"=w1071:errorcluster)  [unwired: 13 in]
                n305 = call "GEA2 Write ERD.vi"("GEA2 Reference In"=w1076, "GEA Inputs"=w1067, "Write ERD List"=w1070, "Error In"=w1071, "Verify ERD Response?"=TRUE) -> ("GEA2 Reference Out"=w1066:refnum<k24>, "Error Out"=w1077:errorcluster)  [unwired: 8 in, 1 out]
              }
            }
          }
          event "Clear Fault Table Buffer": Value Change {
            n306 = event-data() -> ()  [unwired: 1 in, 6 out]
            n307 = Bundle By Name(cluster=T28 {"ERD Number"=130, "Data Type"=enum."string", "Data"=""} ("ERD Read Data In"), "Data"="FF") -> (w1096:T28)
            n308 = Build Array(w1096) -> (w1090:T28[])
            n309 = call "Convert Write ERD List to Message.vi"("GEA Inputs"=w1087, "Write ERD List"=w1090, "Error In"=w1086) -> ("GEA Message"=w1092:T5, "Error Out"=w1093:errorcluster)  [unwired: 11 in]
            n310 = call "GEA2MessageFormatter.vi"("Prefix(Send/Recv)"="SEND", "GEA2 Data In"=w1092, "Error In"=w1093) -> ("Output String"=w1094:string, "Error Out"=w1095:errorcluster)  [unwired: 11 in]
            n311 = call "GExplorer_Queue_GEA2.vi"("Output String"=w1094, "error in (no error)"=w1095) -> ("error out"=w1091:errorcluster)  [unwired: 13 in]
            n312 = call "GEA2 Write ERD.vi"("GEA2 Reference In"=w1085, "Read Timeout (ms)"=u32 2000, "GEA Inputs"=w1087, "Write ERD List"=w1090, "Error In"=w1091, "Verify ERD Response?"=FALSE) -> ("GEA2 Reference Out"=w1084:refnum<k24>, "Error Out"=w1083:errorcluster)  [unwired: 7 in, 1 out]
          }
          event "Clear Cycle Buffer": Value Change {
            n313 = event-data() -> ()  [unwired: 1 in, 6 out]
            n314 = Build Array(T28 {"ERD Number"=136, "Data Type"=enum."string", "Data"="FF"} ("ERD Read Data In")) -> (w1110:T28[])
            n315 = call "Convert Write ERD List to Message.vi"("GEA Inputs"=w1105, "Write ERD List"=w1110, "Error In"=w1108) -> ("GEA Message"=w1112:T5, "Error Out"=w1113:errorcluster)  [unwired: 11 in]
            n316 = call "GEA2MessageFormatter.vi"("Prefix(Send/Recv)"="SEND", "GEA2 Data In"=w1112, "Error In"=w1113) -> ("Output String"=w1114:string, "Error Out"=w1115:errorcluster)  [unwired: 11 in]
            n317 = call "GExplorer_Queue_GEA2.vi"("Output String"=w1114, "error in (no error)"=w1115) -> ("error out"=w1111:errorcluster)  [unwired: 13 in]
            n318 = call "GEA2 Write ERD.vi"("GEA2 Reference In"=w1107, "GEA Inputs"=w1105, "Write ERD List"=w1110, "Error In"=w1111) -> ("Error Out"=w1104:errorcluster)  [unwired: 9 in, 2 out]
            n319 = call "Time Delay6"("error in (no error)"=w1104) -> ("error out"=w1099:errorcluster)  [unwired: 10 in]
            n320 = property on="Get Cycle History" class="Bool (strict)"(error in=w1099, "Val(Sgnl)"=TRUE ("Get Cycle History")) -> (error out=w1103:errorcluster)  [unwired: 1 in, 1 out]
            n321 = call "Time Delay7"("error in (no error)"=w1103) -> ("error out"=w1098:errorcluster)  [unwired: 10 in]
            n322 = property on="Get Cycle History" class="Bool (strict)"(error in=w1098, "Val(Sgnl)"=FALSE ("Get Cycle History")) -> (error out=w1102:errorcluster)  [unwired: 1 in, 1 out]
          }
          event "Get Cycle History": Value Change {
            w1122 = T8[] [{"ERD Number"=135, "Data Type"=enum."string"}, {"ERD Number"=57344, "Data Type"=enum."string"}, {"ERD Number"=57345, "Data Type"=enum."string"}, {"ERD Number"=57346, "Data Type"=enum."string"}, {"ERD Number"=57347, "Data Type"=enum."string"}, {"ERD Number"=57348, "Data Type"=enum."string"}, {"ERD Number"=57349, "Data Type"=enum."string"}, {"ERD Number"=57350, "Data Type"=enum."string"}, {"ERD Number"=57351, "Data Type"=enum."string"}, {"ERD Number"=57352, "Data Type"=enum."string"}, {"ERD Number"=57353, "Data Type"=enum."string"}] ("Read ERD List")
            n323 = event-data() -> ()  [unwired: 1 in, 6 out]
            n324 = call "Convert Read ERD List to Message.vi"("GEA Inputs"=w1117, "Read ERD List"=w1122, "Error In"=w1124) -> ("GEA Message"=w1128:T5, "Error Out"=w1129:errorcluster)  [unwired: 11 in]
            n325 = call "GEA2MessageFormatter.vi"("Prefix(Send/Recv)"="SEND", "GEA2 Data In"=w1128, "Error In"=w1129) -> ("Output String"=w1127:string, "Error Out"=w1126:errorcluster)  [unwired: 11 in]
            n326 = call "GExplorer_Queue_GEA2.vi"("Output String"=w1127, "error in (no error)"=w1126) -> ("error out"=w1123:errorcluster)  [unwired: 13 in]
            n327 = call "GEA2 Read ERD Multiple Messages.vi"("GEA2 Reference In"=w1118, "Read Timeout (ms)"=u32 500, "GEA Inputs"=w1117, "Read ERD List"=w1122, "Error In"=w1123, "#ERDs per message"=4, "Verify ERD Response?"=TRUE) -> ("ERD Data Out"=w1130:T33[], "Error Out"=w1121:errorcluster)  [unwired: 5 in, 2 out]
            n328 = call "Cycle_Diag_Table_Read_TL24.vi"("ERD Data In"=w1130, "error in (no error)"=w1121) -> ("Cycle Buffer Status"=→"Cycle Buffer Status":T16, "Diag Cycle String Out"=→"Diagnostics Table":string[][], "error out"=w1116:errorcluster)  [unwired: 10 in, 1 out]
          }
          event "Save Cycle History Log": Value Change {
            w1138 = T8[] [{"ERD Number"=135, "Data Type"=enum."string"}, {"ERD Number"=57344, "Data Type"=enum."string"}, {"ERD Number"=57345, "Data Type"=enum."string"}, {"ERD Number"=57346, "Data Type"=enum."string"}, {"ERD Number"=57347, "Data Type"=enum."string"}, {"ERD Number"=57348, "Data Type"=enum."string"}, {"ERD Number"=57349, "Data Type"=enum."string"}, {"ERD Number"=57350, "Data Type"=enum."string"}, {"ERD Number"=57351, "Data Type"=enum."string"}, {"ERD Number"=57352, "Data Type"=enum."string"}, {"ERD Number"=57353, "Data Type"=enum."string"}] ("Read ERD List")
            n329 = event-data() -> ()  [unwired: 1 in, 6 out]
            n330 = call "Convert Read ERD List to Message.vi"("GEA Inputs"=w1141, "Read ERD List"=w1138, "Error In"=w1140) -> ("GEA Message"=w1147:T5, "Error Out"=w1148:errorcluster)  [unwired: 11 in]
            n331 = call "GEA2MessageFormatter.vi"("Prefix(Send/Recv)"="SEND", "GEA2 Data In"=w1147, "Error In"=w1148) -> ("Output String"=w1146:string, "Error Out"=w1145:errorcluster)  [unwired: 11 in]
            n332 = call "GExplorer_Queue_GEA2.vi"("Output String"=w1146, "error in (no error)"=w1145) -> ("error out"=w1143:errorcluster)  [unwired: 13 in]
            n333 = call "GEA2 Read ERD Multiple Messages.vi"("GEA2 Reference In"=w1139, "Read Timeout (ms)"=u32 500, "GEA Inputs"=w1141, "Read ERD List"=w1138, "Error In"=w1143, "#ERDs per message"=4, "Verify ERD Response?"=TRUE) -> ("ERD Data Out"=w1137:T33[], "Error Out"=w1142:errorcluster)  [unwired: 5 in, 2 out]
            n334 = call "Cycle_Diag_Table_Read_TL24.vi"("ERD Data In"=w1137, "error in (no error)"=w1142) -> ("Diag Cycle String Out"=w1136:string[][], "error out"=w1135:errorcluster)  [unwired: 10 in, 2 out]
            n335 = call "Cycle_History_Logging.vi"("error in (no error)"=w1135, "Diag Cycle String Out"=w1136) -> ("error out"=w1134:errorcluster)  [unwired: 9 in]
          }
          event "Data ON": Value Change {
            n336 = event-data() -> ()  [unwired: 1 in, 6 out]
            n337 = case shown="True" "Data ON" {
              tunnel: w1155 -> [w1158 w1162]
              tunnel: [w1157 w1161] -> w1154
              tunnel: w1152 -> [w1156 w1160]
              frame True {
                n338 = Enqueue Element(queue=w1156, element=T24 {"Data"=variant, "State"=enum."Init"} ("Data"), error in (no error)=w1158) -> (error out=w1157:errorcluster)  [unwired: 1 in, 2 out]
              }
              frame False {
                n339 = Enqueue Element(queue=w1160, element=T24 {"Data"=variant, "State"=enum."Pause"} ("Data"), error in (no error)=w1162) -> (error out=w1161:errorcluster)  [unwired: 1 in, 2 out]
              }
            }
          }
          event "Stop": Value Change; User Event; Panel Close {
            n340 = event-data() -> ()  [unwired: 1 in, 3 out]
            n341 = call "Control_ERD_Loop_Brass.vi"("Command (ERD Loop Control)"=ERD_Loop_Control_Command_Brass."Shutdown", "Error In"=w1171) -> ("Error Out"=w1170:errorcluster)  [unwired: 13 in]
            n342 = call "Control_GEA2_Loop_Brass.vi"("Command (ERD Loop Control)"=GEA2_Control_Command_Brass."Shutdown", "Error In"=w1170) -> ("Error Out"=w1172:errorcluster)  [unwired: 13 in]
            n343 = call "Control_Cont_Send_Brass.vi"("Command (ERD Loop Control)"=GEA2_Control_Command_Brass."Shutdown", "Error In"=w1172) -> ("Error Out"=w1166:errorcluster)  [unwired: 13 in]
            n344 = call "Time Delay"("error in (no error)"=w1166, "Delay Time (s)"=2.0) -> ("error out"=w1165:errorcluster)  [unwired: 9 in]
          }
        }
        n345 = call "Error_Control_Brass.vi"("Error In"=w422) -> ("Error Out"=w424:errorcluster)  [unwired: 14 in]
      }
      n346 = Unbundle By Name(T24 {"Data"=variant, "State"=enum."Init"} ("Data")) -> ("State"=w65:T25)
      n347 = Build Array(w28, w61, w59, w60, w27, w26, w25, w24) -> (w58:refnum<vi>[])
      n348 = while "Periodic ERD Query Loop" {
        shift-right: [w180] -> w55
        shift-left: w73 -> [w182]
        tunnel: w63 -> [w183]
        shift-right: [w177] -> _
        shift-left: _ -> [w176]
        shift-right: [w171] -> _
        shift-left: w65 -> [w173]
        shift-right: [w166] -> _
        shift-left: _ -> [w165]
        tunnel: w62 -> [w164]
        tunnel: [w163] -> w53
        shift-right: [w162] -> _
        shift-left: _ -> [w161]
        tunnel: w58 -> [w160]
        i -> [w159]
        stop <- w179 stop-if-true
        # "ERD Loop"
        n349 = Dequeue Element(queue=w183, timeout in ms (-1)=0, error in (no error)=w182) -> (element=w168:T24, timed out?=w174:bool, error out=w181:errorcluster)  [unwired: 1 out]
        n350 = Unbundle By Name(w168) -> ("State"=w158:T25)
        n351 = Select(t=w173, s=w174, f=w158) -> (s? t:f=w172:T25)
        n352 = call "FGV_GEA2_Ref.vi"("Action"=enum16{"Set Ref", "Get Ref"}."Get Ref", "Error In"=w181) -> ("GEA2 Reference Out"=w167:refnum<k24>, "Error Out"=w170:errorcluster)  [unwired: 12 in]
        n353 = case shown="\"Read ERDs\"" w172 {
          tunnel: w170 -> [w193 w201 w214 w228 w248 w289 w336 w364 w372]
          tunnel: [w185 w197 w207 w228 w246 w288 w333 w364 w372] -> w178
          tunnel: [_ _ _ _ _ _ _ _ TRUE] -> w179
          tunnel: [w192 w199 w205 w231 w252 w282 w343 w365 w370] -> w177
          tunnel: w176 -> [w192 w199 w226 w231 w252 w282 w343 w365 w370]
          tunnel: T7 {"Source"=229, "Destination"=60} ("GEA Inputs") -> [_ _ w203 _ w236 w286 _ _ _]
          tunnel: [ERD_Loop_States_Brass."Build ERD Read List" ("State") ERD_Loop_States_Brass."Read ERDs" ("State") ERD_Loop_States_Brass."Update UI" ("State") ERD_Loop_States_Brass."Update Graphs" ("State") ERD_Loop_States_Brass."Read Faults" ("State") ERD_Loop_States_Brass."Log Data" ("State") ERD_Loop_States_Brass."Read ERDs" ("State") ERD_Loop_States_Brass."Pause" ("State") ERD_Loop_States_Brass."Shutdown" ("State")] -> w171
          tunnel: w167 -> [_ _ w215 _ w241 w287 _ _ _]
          tunnel: [w190 w200 w204 w233 w250 w283 w342 w362 w368] -> w166
          tunnel: w165 -> [w190 _ w204 w233 w250 w283 w342 w362 w368]
          tunnel: w164 -> [w189 w196 w212 w229 w249 w281 w341 w361 w367]
          tunnel: [w189 w196 w212 w229 w249 w281 w340 w361 w367] -> w163
          tunnel: [w188 w195 w206 w230 w240 w284 w319 w360 w366] -> w162
          tunnel: w161 -> [w188 w195 _ w230 w238 w285 w319 w360 w366]
          tunnel: w160 -> [_ _ _ _ w242 _ _ _ _]
          tunnel: w159 -> [_ _ _ _ _ _ _ _ _]
          frame "Init", Default {
            # "Set Write Header\nFGV to True"
            n354 = call "Write_Header_FGV.vi"("Write Header ? In"=TRUE, "Action"=enum16{"Get", "Set"}."Set", "Error In"=w193) -> ("Error Out"=w185:errorcluster)  [unwired: 11 in, 1 out]
          }
          frame "Build ERD Read List" {
            n355 = call "ERD_Read_List_Builder.vi"("Array"="ERD Read List", "Error In"=w201) -> ("Read ERD List"=w200:T8[], "Error Out"=w197:errorcluster)  [unwired: 16 in]
          }
          frame "Read ERDs" {
            n356 = call "Convert Read ERD List to Message.vi"("GEA Inputs"=w203, "Read ERD List"=w204, "Error In"=w214) -> ("GEA Message"=w223:T5, "Error Out"=w224:errorcluster)  [unwired: 11 in]
            n357 = call "GEA2MessageFormatter.vi"("Prefix(Send/Recv)"="SEND", "GEA2 Data In"=w223, "Error In"=w224) -> ("Output String"=w222:string, "Error Out"=w221:errorcluster)  [unwired: 11 in]
            n358 = call "GExplorer_Queue_GEA2.vi"("Output String"=w222, "error in (no error)"=w221) -> ("error out"=w219:errorcluster)  [unwired: 13 in]
            n359 = Tick Count (ms)() -> (millisecond timer value=w205:u32)
            n360 = Subtract(x=w205, y=w226) -> (x-y=→"Log Rate (ms)":u32)
            n361 = call "GEA2 Read ERD Multiple Messages.vi"("GEA2 Reference In"=w215, "Retry Count"=1, "Read Timeout (ms)"=u32 200, "GEA Inputs"=w203, "Read ERD List"=w204, "Error In"=w219, "#ERDs per message"=7, "Verify ERD Response?"=FALSE) -> ("ERD Data Out"=w202:T33[], "Error Out"=w211:errorcluster)  [unwired: 4 in, 2 out]
            n362 = call "Write_Header_FGV.vi"("Action"=enum16{"Get", "Set"}."Get", "Error In"=w211) -> ("Write Header ? Out"=w208:bool, "Error Out"=w210:errorcluster)  [unwired: 12 in]
            n363 = call "Convert_ERDs_Brass.vi"("New Header?"=w208, "Array"=w202, "Error In"=w210) -> ("All_ERD_Data_Bundled_Brass"=w206:T34, "Error Out"=w207:errorcluster)  [unwired: 11 in]
          }
          frame "Update UI" {
            n364 = Unbundle By Name(w230) -> ("Version"=→"Version":T6, "ERD_Always Show"=→"ERD_Always Show":T1)
          }
          frame "Update Graphs" {
            n365 = case shown="True" "ERD Graphing ON" {
              tunnel: w248 -> [w270 w278]
              tunnel: [w270 w277] -> w247
              tunnel: "ERD Graph Cntrl" -> [_ w276]
              tunnel: [_ w275] -> w243
              tunnel: w241 -> [_ w274]
              tunnel: w238 -> [w269 w273]
              tunnel: [w269 w272] -> w237
              tunnel: w236 -> [_ w271]
              frame False {
              }
              frame True {
                n366 = call "Graph ERD Read List_Brass.vi"("GEA2 Reference In"=w274, "GEA Inputs"=w271, "All_Bundled_Data_Brass"=w273, "ERD Graph Cntrl"=w276, "Error In"=w278) -> ("ERD Graph  Ind"=w275:T11, "All_Bundled_Data_Brass 2"=w272:T34, "Error Out"=w277:errorcluster)  [unwired: 7 in, 1 out]
              }
            }
            n367 = case shown="True" "Graphing ON" {
              tunnel: w247 -> [w253 w268]
              tunnel: [w253 w267] -> w246
              tunnel: w243 -> [_ w265]
              tunnel: w242 -> [_ w260]
              tunnel: w237 -> [w254 w259]
              tunnel: [w254 w259] -> w240
              frame False {
              }
              frame True {
                n368 = call "Update Graphs_Brass.vi"("Select Graph"="Select Graph", "appended array"=w260, "ERD Graph  Ind 2"=w265, "All_Bundled_Data_Brass"=w259, "Error In"=w268) -> ("Dryer Loads"=→"Dryer Loads":dbl[][], "Washer Loads"=→"Washer Loads":u16[][], "Water Temperature"=→"Water Temperature":dbl, "Basket Speed"=→"Basket Speed":u16, "Pressure"=→"Pressure 2":dbl, "ERD 3"=→"ERD 3":dbl, "ERD 2"=→"ERD 2":dbl, "ERD 1"=→"ERD 1":dbl, "Error Out"=w267:errorcluster)  [unwired: 2 in]
                "ERD Graph  Ind" <- w265
              }
            }
          }
          frame "Read Faults" {
            n369 = case shown="True" "Fault ON" {
              tunnel: w289 -> [w290 w299]
              tunnel: [w290 w298] -> w288
              tunnel: w287 -> [_ w297]
              tunnel: w286 -> [_ w296]
              tunnel: w285 -> [w291 w295]
              tunnel: [w291 w294] -> w284
              frame False {
              }
              frame True {
                # "0-11 Sequence\n12-20 Table"
                n370 = call "GEA2 Read ERD Multiple Messages.vi"("GEA2 Reference In"=w297, "Retry Count"=2, "Read Timeout (ms)"=u32 250 ("Read Timeout (ms) 2"), "GEA Inputs"=w296, "Read ERD List"=T8[] [{"ERD Number"=132, "Data Type"=enum."string"}, {"ERD Number"=141, "Data Type"=enum."uint32_t"}, {"ERD Number"=57394, "Data Type"=enum."string"}, {"ERD Number"=57395, "Data Type"=enum."string"}, {"ERD Number"=57396, "Data Type"=enum."string"}, {"ERD Number"=57397, "Data Type"=enum."string"}, {"ERD Number"=57398, "Data Type"=enum."string"}, {"ERD Number"=57399, "Data Type"=enum."string"}, {"ERD Number"=57400, "Data Type"=enum."string"}, {"ERD Number"=57401, "Data Type"=enum."string"}, {"ERD Number"=57402, "Data Type"=enum."string"}, {"ERD Number"=57403, "Data Type"=enum."string"}, {"ERD Number"=129, "Data Type"=enum."string"}, {"ERD Number"=57444, "Data Type"=enum."string"}, {"ERD Number"=57445, "Data Type"=enum."string"}, {"ERD Number"=57446, "Data Type"=enum."string"}, {"ERD Number"=57447, "Data Type"=enum."string"}, {"ERD Number"=57448, "Data Type"=enum."string"}, {"ERD Number"=57449, "Data Type"=enum."string"}, {"ERD Number"=57450, "Data Type"=enum."string"}, {"ERD Number"=57451, "Data Type"=enum."string"}], "Error In"=w299, "#ERDs per message"=5 ("#ERDs per message 2"), "Verify ERD Response?"=FALSE) -> ("ERD Data Out"=w304:T33[], "Error Out"=w298:errorcluster)  [unwired: 4 in, 2 out]
                n371 = Array Subset(array=w304, index=12, length=11) -> (w305:T33[])
                n372 = Array Subset(array=w304, index=0, length=12) -> (w303:T33[])
                n373 = call "Fault_Table_Read.vi"("ERD Data Out"=w305) -> ("Fault Set?"=→"Fault Status":bool, "Table Buffer Status"=→"Table Buffer Status":T15, "Fault Table String Out"=→"Fault Table Buffer":string[][], "Fault Table Array Out"=w293:T36)  [unwired: 11 in]
                n374 = call "Fault_Seq_Read.vi"("Seq ERD In"=w303) -> ("Seq Buffer Status"=→"Seq Buffer Status":T15, "String"=→"Fault Sequence Buffer":string)  [unwired: 13 in]
                n375 = Bundle By Name(cluster=w295, "Fault Table Array"=w293) -> (w294:T34)
              }
            }
          }
          frame "Log Data" {
            # "TimeStamp"
            # "Append With Fault Log Data"
            # "Write Date/Time Header"
            n376 = Unbundle By Name(w319) -> ("CSV File String Arrays.ERD Name Array"=w339:string[], "CSV File String Arrays.ERD Number Array"=w338:string[], "CSV File String Arrays.ERD Converted String Data"=w331:string[])
            n377 = call "Write_Header_FGV.vi"("Action"=enum16{"Get", "Set"}."Get", "Error In"=w336) -> ("Write Header ? Out"=w317:bool, "Error Out"=w330:errorcluster)  [unwired: 12 in]
            n378 = case shown="True" w317 {
              tunnel: w339 -> [w352 _]
              tunnel: [w354 string[] [] ("ERD Name Array")] -> w329
              tunnel: w338 -> [w353 _]
              tunnel: [w357 string[] [] ("ERD Number Array")] -> w327
              frame True {
                n379 = Insert Into Array(array=w353, index=0, new element #1="", new element #2="", new element #3="", new element #4="") -> (w357:string[])
                n380 = Insert Into Array(array=w352, index=0, new element #1="Date", new element #2="Time", new element #3="HH:MM:SS", new element #4=".SS" ("new element/subarray")) -> (w354:string[])
              }
              frame False {
              }
            }
            n381 = call "TimeStamp to String Array.vi"("String Array In"=w331) -> ("String Array Out"=w325:string[])  [unwired: 10 in]
            n382 = Unbundle By Name(w319) -> ("Fault Table Array"=w318:T36)
            n383 = call "Faults_To_String_Array.vi"("Write Header ?"=w317, "Fault Table Entry"=w318, "Error In"=w330) -> ("Fault Header String Array"=w324:string[], "Fault ERD Number String Array"=w323:string[], "Fault Data String Array"=w322:string[], "Error Out"=w320:errorcluster)  [unwired: 13 in]
            n384 = Insert Into Array(array=w329, new element=w324) -> (w328:string[])  [unwired: 1 in]
            n385 = Insert Into Array(array=w327, new element=w323) -> (w326:string[])  [unwired: 1 in]
            n386 = Insert Into Array(array=w325, new element=w322) -> (w321:string[])  [unwired: 1 in]
            n387 = call "Write _To_CSV_File.vi"("Refnum In"=w341, "String Array 1"=w328, "String Array 2"=w326, "String Array 3"=w321, "Error In"=w320) -> ("Refnum Out"=w340:refnum<file>, "Error Out"=w334:errorcluster)  [unwired: 12 in, 1 out]
            n388 = call "Write_Header_FGV.vi"("Write Header ? In"=FALSE, "Action"=enum16{"Get", "Set"}."Set", "Error In"=w334) -> ("Error Out"=w333:errorcluster)  [unwired: 11 in, 1 out]
          }
          frame "Pause" {
          }
          frame "Shutdown" {
          }
        }
        n389 = call "Error_Control_Brass.vi"("Error In"=w178) -> ("Error Out"=w180:errorcluster)  [unwired: 14 in]
      }
      n390 = while "GEA2 Receive Message Loop" {
        shift-right: [w1178] -> w119
        shift-left: w38 -> [w1179]
        shift-right: [w1175] -> _
        shift-left: w108 -> [w1180]
        stop <- w1177 stop-if-true
        # "GEA2 Receive Message Loop"
        n391 = event shown="[0] <Data>: User Event" {
          selector: w1180 -> [w1196 w1198 w1214 w1220]
          dyn-events: [w1196 w1198 w1209 w1220] -> w1175
          timeout: _ -> [_ _ _ _]
          tunnel: w1179 -> [w1195 w1200 w1217 w1222]
          tunnel: [w1183 w1200 w1202 w1222] -> w1176
          tunnel: [FALSE TRUE _ TRUE] -> w1177
          event User Event {
            n392 = event-data() -> ("Source"=w1190:u8, "Destination"=w1189:u8, "Command"=w1188:u8, "Message"=w1187:string)  [unwired: 1 in]
            n393 = Bundle By Name(cluster=T5 {"Source"=0, "Destination"=0, "Command"=0, "Message"=""} ("GEA2 Msg"), "Source"=w1190, "Destination"=w1189, "Command"=w1188, "Message"=w1187) -> (w1181:T5)
            n394 = call "GEA2 Log Filter.vi"("Filter Log"="Filter Log", "Filter Data"="Filter Data", "GEA2 Msg"=w1181, "Cmd to Filter"="Cmd", "error in (no error)"=w1195) -> ("error out"=w1184:errorcluster)  [unwired: 10 in]
            n395 = call "FGV_GEA2_Ref.vi"("Action"=enum16{"Set Ref", "Get Ref"}."Get Ref", "Error In"=w1184) -> ("GEA2 Reference Out"=w1182:refnum<k24>, "Error Out"=w1185:errorcluster)  [unwired: 12 in]
            n396 = call "ACK Subscriptions Publications.vi"("GEA2 Reference In"=w1182, "GEA2 Msg"=w1181, "error in (no error)"=w1185) -> ("error out"=w1183:errorcluster)  [unwired: 11 in, 1 out]
          }
          event User Event {
            n397 = event-data() -> ()  [unwired: 1 in, 1 out]
          }
          event "Board Index": Value Change {
            # "Stop old GEA2\nbus reference"
            # "Allow other references a chance\nto begin using new reference"
            # "Store new GEA2 bus reference"
            # "Update event registration\nand initialize new GEA2 bus"
            # "Get the previous GEA2\nbus ref, but don't stop it\nuntil we update the FGV\nwith the new GEA2 ref"
            n398 = event-data() -> ("NewVal"=w1213:u8)  [unwired: 1 in]
            n399 = property on="Board Index" class="DigNum (strict)"(error in=w1217, "DisabledEnum"=T29."Disabled and Grayed Out" ("Disabled")) -> (error out=w1218:errorcluster)  [unwired: 1 in, 1 out]
            n400 = call "FGV_GEA2_Ref.vi"("Action"=enum16{"Set Ref", "Get Ref"}."Get Ref", "Error In"=w1218) -> ("GEA2 Reference Out"=w1201:refnum<k24>, "Error Out"=w1215:errorcluster)  [unwired: 12 in]
            n401 = call "GEA2_Reregister.vi"("Board Index"=w1213, "Event Registration In"=w1214, "Error In"=w1215) -> ("GEA2 Reference Out"=w1207:refnum<k24>, "Board ID"=w1210:string, "Event Registration Out"=w1209:refnum<event-registration>, "Error Out"=w1211:errorcluster)  [unwired: 9 in]
            n402 = property on="Board Index" class="DigNum (strict)"(error in=w1211, "DisabledEnum"=T29."Enabled" ("Disabled")) -> (error out=w1208:errorcluster)  [unwired: 1 in, 1 out]
            n403 = local write "Board ID"(w1210) -> ()
            n404 = call "FGV_GEA2_Ref.vi"("GEA2 Reference In"=w1207, "Action"=enum16{"Set Ref", "Get Ref"}."Set Ref", "Error In"=w1208) -> ("Error Out"=w1204:errorcluster)  [unwired: 11 in, 1 out]
            n405 = call "Time Delay"("error in (no error)"=w1204, "Delay Time (s)"=3.0) -> ("error out"=w1203:errorcluster)  [unwired: 9 in]
            n406 = call "GEA2 Stop.vi"("GEA2 Reference In"=w1201, "Error In"=w1203) -> ("Error Out"=w1202:errorcluster)  [unwired: 13 in]
          }
          event "Stop": Value Change {
            n407 = event-data() -> ()  [unwired: 1 in, 6 out]
          }
        }
        n408 = call "Error_Control_Brass.vi"("Error In"=w1176) -> ("Error Out"=w1178:errorcluster)  [unwired: 14 in]
      }
      n409 = while "Continuous Send Loop" {
        shift-right: [w133] -> _
        shift-left: Cont_Send_States."Run" ("State") -> [w132]
        tunnel: w43 -> [w134]
        tunnel: [w127] -> _
        shift-right: [w125] -> w47
        shift-left: w38 -> [w136]
        stop <- w135 stop-if-true
        # "Continuous Send Loop"
        n410 = Dequeue Element(queue=w134, timeout in ms (-1)=0, error in (no error)=w136) -> (queue out=w128:refnum<queue>, element=w121:T21, timed out?=w129:bool, error out=w124:errorcluster)
        n411 = Select(t=w132, s=w129, f=w121) -> (s? t:f=w131:T21)
        n412 = property on="GEA2 Send" class="Clust (strict)"() -> ("Value"=w123:T5)  [unwired: 2 in, 2 out]
        n413 = case shown="\"Run\", Default" w131 {
          selector: w131 -> [w140 w155]
          tunnel: w124 -> [w142 w157]
          tunnel: [w141 w157] -> w126
          tunnel: [_ TRUE] -> w135
          tunnel: [w140 w155] -> w133
          tunnel: w128 -> [w139 w154]
          tunnel: [w139 w154] -> w127
          tunnel: w123 -> [w138 _]
          frame "Run", Default {
            n414 = case shown="True" "Start Send" {
              tunnel: w142 -> [w143 w146]
              tunnel: [w143 w150] -> w141
              tunnel: w138 -> [_ w148]
              frame False {
              }
              frame True {
                n415 = call "FGV_GEA2_Ref.vi"("Action"=enum16{"Set Ref", "Get Ref"}."Get Ref", "Error In"=w146) -> ("GEA2 Reference Out"=w144:refnum<k24>, "Error Out"=w145:errorcluster)  [unwired: 12 in]
                n416 = call "GEA2MessageFormatter.vi"("Prefix(Send/Recv)"="SEND", "GEA2 Data In"=w148, "Error In"=w145) -> ("Output String"=w149:string, "Error Out"=w153:errorcluster)  [unwired: 11 in]
                n417 = call "GExplorer_Queue_GEA2.vi"("Output String"=w149, "error in (no error)"=w153) -> ("error out"=w151:errorcluster)  [unwired: 13 in]
                n418 = call "GEA2 Send Message.vi"("GEA2 Reference In"=w144, "Input Data"=w148, "Error In"=w151) -> ("Error Out"=w150:errorcluster)  [unwired: 11 in, 1 out]
              }
            }
          }
          frame "Shutdown" {
          }
        }
        n419 = call "Error_Control_Brass.vi"("Error In"=w126) -> ("Error Out"=w125:errorcluster)  [unwired: 14 in]
        n420 = Wait (ms)(milliseconds to wait="Msg Rate (ms)") -> ()  [unwired: 1 out]
      }
      n421 = while "GEA2 Display Loop" {
        tunnel: w64 -> [w382]
        shift-right: [w379] -> _
        shift-left: _ -> [w385]
        shift-right: [w381] -> w90
        shift-left: w37 -> [w389]
        tunnel: w35 -> [w375]
        tunnel: [w373] -> w33
        stop <- w383 stop-if-true
        # "GEA2 Display Loop"
        n422 = Dequeue Element(queue=w382, error in (no error)=w389) -> (element=w388:T23, error out=w384:errorcluster)  [unwired: 1 in, 2 out]
        n423 = Unbundle By Name(w388) -> ("Data"=w386:variant, "State"=w387:enum16{"Add to Log", "Clear", "Shutdown"})
        n424 = case shown="\"Add to Log\", Default" w387 {
          tunnel: w386 -> [w400 _ _]
          tunnel: w385 -> [w403 w408 _]
          tunnel: [w402 w408 ""] -> w380
          tunnel: w384 -> [w401 w409 w413]
          tunnel: [w398 w409 w413] -> w376
          tunnel: [FALSE TRUE FALSE] -> w383
          tunnel: [w390 _ _] -> w374
          frame "Add to Log", Default {
            n425 = Variant To Data(error in=w401, type="", Variant=w400) -> (data=w392:string, error out=w398:errorcluster)
            n426 = String Subset(string=w392, offset (0)=22, length (rest)=7 ("length (rest)")) -> (substring=w393:string)
            n427 = Equal?(x="SEND E5", y=w393) -> (x = y?=w391:bool)
            n428 = case shown="True" w391 {
              tunnel: w403 -> [w406 w407]
              tunnel: [w405 w407] -> w402
              tunnel: w392 -> [w404 _]
              tunnel: [w404 _] -> w390
              frame False {
                n429 = Concatenate Strings(w404, w406) -> (w405:string)
              }
              frame True {
              }
            }
          }
          frame "Shutdown" {
          }
          frame "Clear" {
          }
        }
        "GEA2 Log" <- w380
        n430 = call "Write _To_TXT_File.vi"("refnum"=w375, "text"=w374, "error in"=w376) -> ("refnum out"=w373:refnum<file>, "error out"=w377:errorcluster)  [unwired: 10 in, 1 out]
        n431 = call "Error_Control_Brass.vi"("Error In"=w377) -> ("Error Out"=w381:errorcluster)  [unwired: 14 in]
        n432 = String Subset(string=w380, length (rest)="GEA2 Log Length") -> (substring=w379:string)  [unwired: 1 in]
      }
      n433 = Close File(refnum=w33, error in=w90) -> (error out=w34:errorcluster)  [unwired: 1 out]
      n434 = call "GEA2 Stop.vi"("GEA2 Reference In"=w117, "Error In"=w118) -> ("Error Out"=w101:errorcluster)  [unwired: 13 in]
      n435 = Close File(refnum=w53, error in=w55) -> (error out=w54:errorcluster)  [unwired: 1 out]
      n436 = Merge Errors(w54, w34, w47, w119, w101) -> (w29:errorcluster)
      n437 = Obtain Queue(name (unnamed)="Continuous Send", element data type=Cont_Send_States_Brass."Run" ("State"), error in (no error)=w29) -> (queue out=w52:refnum<queue>, error out=w51:errorcluster)  [unwired: 2 in, 1 out]
      n438 = Obtain Queue(name (unnamed)="ERD Loop", element data type=T24 {"Data"=variant, "State"=enum."Read ERDs"} ("Data"), error in (no error)=w29) -> (queue out=w97:refnum<queue>, error out=w96:errorcluster)  [unwired: 2 in, 1 out]
      n439 = Obtain Queue(name (unnamed)="GEA2", element data type=T23 {"Data"=variant, "State"=enum."Add to Log"} ("Data"), error in (no error)=w29) -> (queue out=w105:refnum<queue>, error out=w104:errorcluster)  [unwired: 2 in, 1 out]
      n440 = Obtain Queue(name (unnamed)="DAQ", element data type=DAQ_States_Brass."Wait for Init" ("States"), error in (no error)=w29) -> (queue out=w92:refnum<queue>, error out=w93:errorcluster)  [unwired: 2 in, 1 out]
      n441 = Release Queue(queue=w52, error in (no error)=w51) -> (error out=w50:errorcluster)  [unwired: 1 in, 2 out]
      n442 = Release Queue(queue=w97, error in (no error)=w96) -> (error out=w86:errorcluster)  [unwired: 1 in, 2 out]
      n443 = Release Queue(queue=w105, error in (no error)=w104) -> (error out=w87:errorcluster)  [unwired: 1 in, 2 out]
      n444 = Release Queue(queue=w92, error in (no error)=w93) -> (error out=w88:errorcluster)  [unwired: 1 in, 2 out]
      n445 = Merge Errors(w50, w86, w87, w88) -> (w85:errorcluster)
      n446 = call "Error_Control_Brass.vi"("Command (Handle Errors)"=Error_Command_Brass."Report Errors", "Error In"=w85) -> ("Error Out"=w79:errorcluster)  [unwired: 13 in]
    }
    frame Error {
    }
  }
  n447 = call <vilib>:"Simple Error Handler.vi"("error in (no error)"=w5) -> ("error out"=→"Error Out":errorcluster)  [unwired: 4 in, 4 out]
